vi "Text control 2 v3.1.vi"() -> ()   [LabVIEW 2016]
panel:
  out "I vs Vd":cluster{"Y data in":dbl[], "X data in":dbl[]}[](graph)
  in  "Auto Reset":bool
  in  "Reset":bool
  out "Id min vs time":cluster{"Y data in":dbl[], "X data in":dbl[]}[](graph)
  in  "Time Offset":dbl caption="Set Start Time (s)"
  out "Total lines":i32
  out "Line running":i32
  in  "byte count":u32=64
  in  "Serial Settings:Serial End Mode for Reads":u16(ring)=2 items=["None", "LastBit", "TermChar"]
  in  "Timeout (ms)":u32=10000
  in  "Enable Termination\nChar (T)":bool=TRUE
  in  "Termination char\n(0xA = '\\n' = LF)\n(0xD = '\\r' = CR)":u8=13 format="%.0x"
  in  "flow control":u16(ring) items=["None"=0, "XON/XOFF"=1, "RTS/CTS"=2, "DTR/DSR"=4]
  in  "stop bits":u16(ring)=10 items=["1.0"=10, "1.5"=15, "2.0"=20]
  in  "parity":u16(ring) items=["None", "Odd", "Even", "Mark", "Space"]
  in  "data bits":u16=8 min=5 max=8 step=1
  in  "VISA resource name":refnum<visa-resource-name>="COM6"
  in  "baud rate":u32=9600
  out "Serial port output":string
  out "error out":errorcluster
  in  "Units":u16(ring) items=["Seconds", "Minutes", "Hours"]
  out "Elapsed Time":dbl caption="Elapsed Time (s)"
  out "Id max vs time":cluster{"Y data in":dbl[], "X data in":dbl[]}[](graph)
  out "Ig":dbl format="%.2e"
  out "Id":dbl format="%.2e"
  out "Is":dbl format="%.2e"
  out "I vs Vg":cluster{"Y data in":dbl[], "X data in":dbl[]}[](graph)
  in  "Panel Controls 2":T1={"Emergency Stop"=refnum, "TransGraph Max"=1e-05, "Text/Graph (text=false)"=TRUE, "TransGraph Min"=1e-11} {"TransGraph Min" format="%.2e"; "TransGraph Max" format="%.2e"}
  out "Command running:":string="#output s 0 0 0 -0.008 0.008 0.002"
  in  "Standby":T2
  in  "Full Reset":bool
  in  "SMU4":cluster{"on/off":bool, "Voltage":dbl} {"Voltage" min=-100.0 max=100.0 format="%.2f"}
  in  "Source/Drain Range":u8(slide)=6 max=11 scale=0.0..11.0
  in  "Source/Drain\nRange mode":u16(ring) items=["Auto", "Limited", "Fixed"]
  in  "Gate Range":u8(slide)=6 max=11 scale=0.0..11.0
  in  "Gate Range\nmode":u16(ring) items=["Auto", "Limited", "Fixed"]
  in  "Gate":T3={"Gate Start"=0.0, "Gate Stop"=2.0, "Gate Step (linear only)"=1.0, "Gate Compliance"=0.0001, "Gate PComp"=0.0, "Range mode"=0, "Range"=6} {"Range" max=11 scale=0.0..11.0; "Range mode" items=["Auto", "Limited", "Fixed"]; "Gate PComp" format="%^.2e"; "Gate Compliance" format="%^.2e"; "Gate Step (linear only)" format="%^.4e"; "Gate Stop" format="%^.4e"; "Gate Start" format="%^.4e"}
  in  "Drain 2":T4={"Drain Start"=0.0, "Drain Stop"=2.0, "Drain Compliance"=0.0001, "Drain Step"=1.0, "Drain PComp"=0.0, "Range mode"=0, "Range"=6} {"Range" max=11 scale=0.0..11.0; "Range mode" items=["Auto", "Limited", "Fixed"]; "Drain PComp" format="%^.2e"; "Drain Step" format="%^.4e"; "Drain Compliance" format="%^.2e"; "Drain Stop" format="%^.4e"; "Drain Start" format="%^.4e"}
  in  "Timings 2":T5={"integration time"=0, "Short/Long integration time"=0.00064, "hold time (sec)"=0.0, "delay time (sec)"=0.0, "Step Time (0 disables)"=0.0, "sweep method"=0, "Pulse period"=0.005, "Base voltage"=0.0, "Pulse width"=0.0005} {"Pulse width" min=0.0005 max=0.1 step=0.0001 format="%.4f"; "Base voltage" format="%^.4e"; "Pulse period" min=0.005 max=1.0 step=0.0001 format="%.4f"; "sweep method" items=["Continuous", "Pulsed"]; "Step Time (0 disables)" format="%.2f"; "delay time (sec)" format="%.4f"; "hold time (sec)" format="%.4f"; "Short/Long integration time" format="%^.0e"; "integration time" scale=0.0..2.0}
  in  "Panel Controls":T6={"Emergency Stop"=refnum, "TransGraph Max"=1e-05, "Text/Graph (text=false)"=TRUE} {"TransGraph Max" format="%.2e"}
  in  "Interrupt run":bool
  in  "Drain: Compliance":dbl=0.001 format="%.8f"
  in  "Gate: Compliance":dbl=0.001 format="%.8f"
  out "Path":path=path "C:/users/rlp38/09Apr2009LTtesting/test2.txt"
  in  "hold time /s":dbl format="%.2f"
  in  "delay time /s":dbl format="%.2f"
  in  "integration time":u32(slide) max=2 step=1 scale=0.0..2.0
  in  "Integration time (short)":dbl=0.0019 min=8e-05 max=0.0019 step=8e-05 format="%^.0e"
  in  "Integration time (long)":dbl=0.32 min=0.04 max=2.0 step=0.02 format="%.2f"
  in  "Step delay /s":dbl format="%.2f"
  in  "Program":string="#pulsedstressV d 0.03 20 0 0.5 0.0827 5\n#\n#itime s\n#gaterangemode l\n#drainrangemode l\n#pulsed on 0.05 0 0.02\n#transfer d 1 -1 -0.1 -1 -1 0\n#wait-min 1\n#transfer d 1 -1 -0.1 -1 -1 0\n#output d 0 -1 -0.5 0 -1 -0.1\n#transfer d -10 40 1 5 40 35\n#transfer d -10 40 1 5 40 35\n#output d 0 40 20 0 40 1\n#\n#\n#sample 1 0.008 221 6 0.003\n#samplei 400e-6 200 6 0.002 0.1\n#vsu2pulse -10 4\n#\n#stressV 0.016 0.03 2e-4 0.1e-3 11\n#stressI 220e-7 0.08 15\n#transfer s -1 1 0.5 -0.005 0.005 0.005\n#output s 0 0 0 -0.008 0.008 0.002\n"
  # "Serial port settings"
  # "Time"
  # "100 samples is approx 13s with medium integration"
  # "Syntax:\nitime [s|m|l]\ngaterangemode [a|l|f]\ndrainrangemode [a|l|f]\npulsed [on|off] PulsePeriod(sec) PulseBaseVoltage PulseONWidth(sec)\nstandby [on l off]\nwait NumMilliseconds\nwait-min NumMinutes\n# texthere = comment\ntransfer [s|d] VgStart VgStop VgStep VdStart VdStop VdStep\noutput [s|d] VgStart VgStop VgStep VdStart VdStop VdStep\nsample Vg Vd NumSamples Time(s) SampleInterval(s)\nsamplei Idg NumSamples Time(s) SampleInterval(s) VDGcompliance\n# if in doubt use SampleInterval(s) = 0.004\nstressV VG VD IGcompliance IDcompliance Duration(sec)\nstressI IDG VDGcompliance Duration(sec)\nvsu2pulse Bias Duration(s)\npulsedstressV [s|d] VEstop VgON VgOFF Period(s) PulseONwidth(s) Vd\nsample-fpp Vg Vd NumSamples Time\nresample-fpp Vg Vd\ntransfer-fpp [s|d] VgStart VgStop VgStep VdStart VdStop VdStep\noutput-fpp [s|d] VgStart VgStop VgStep VdStart VdStop VdStep\nserial SerialPortCommand"
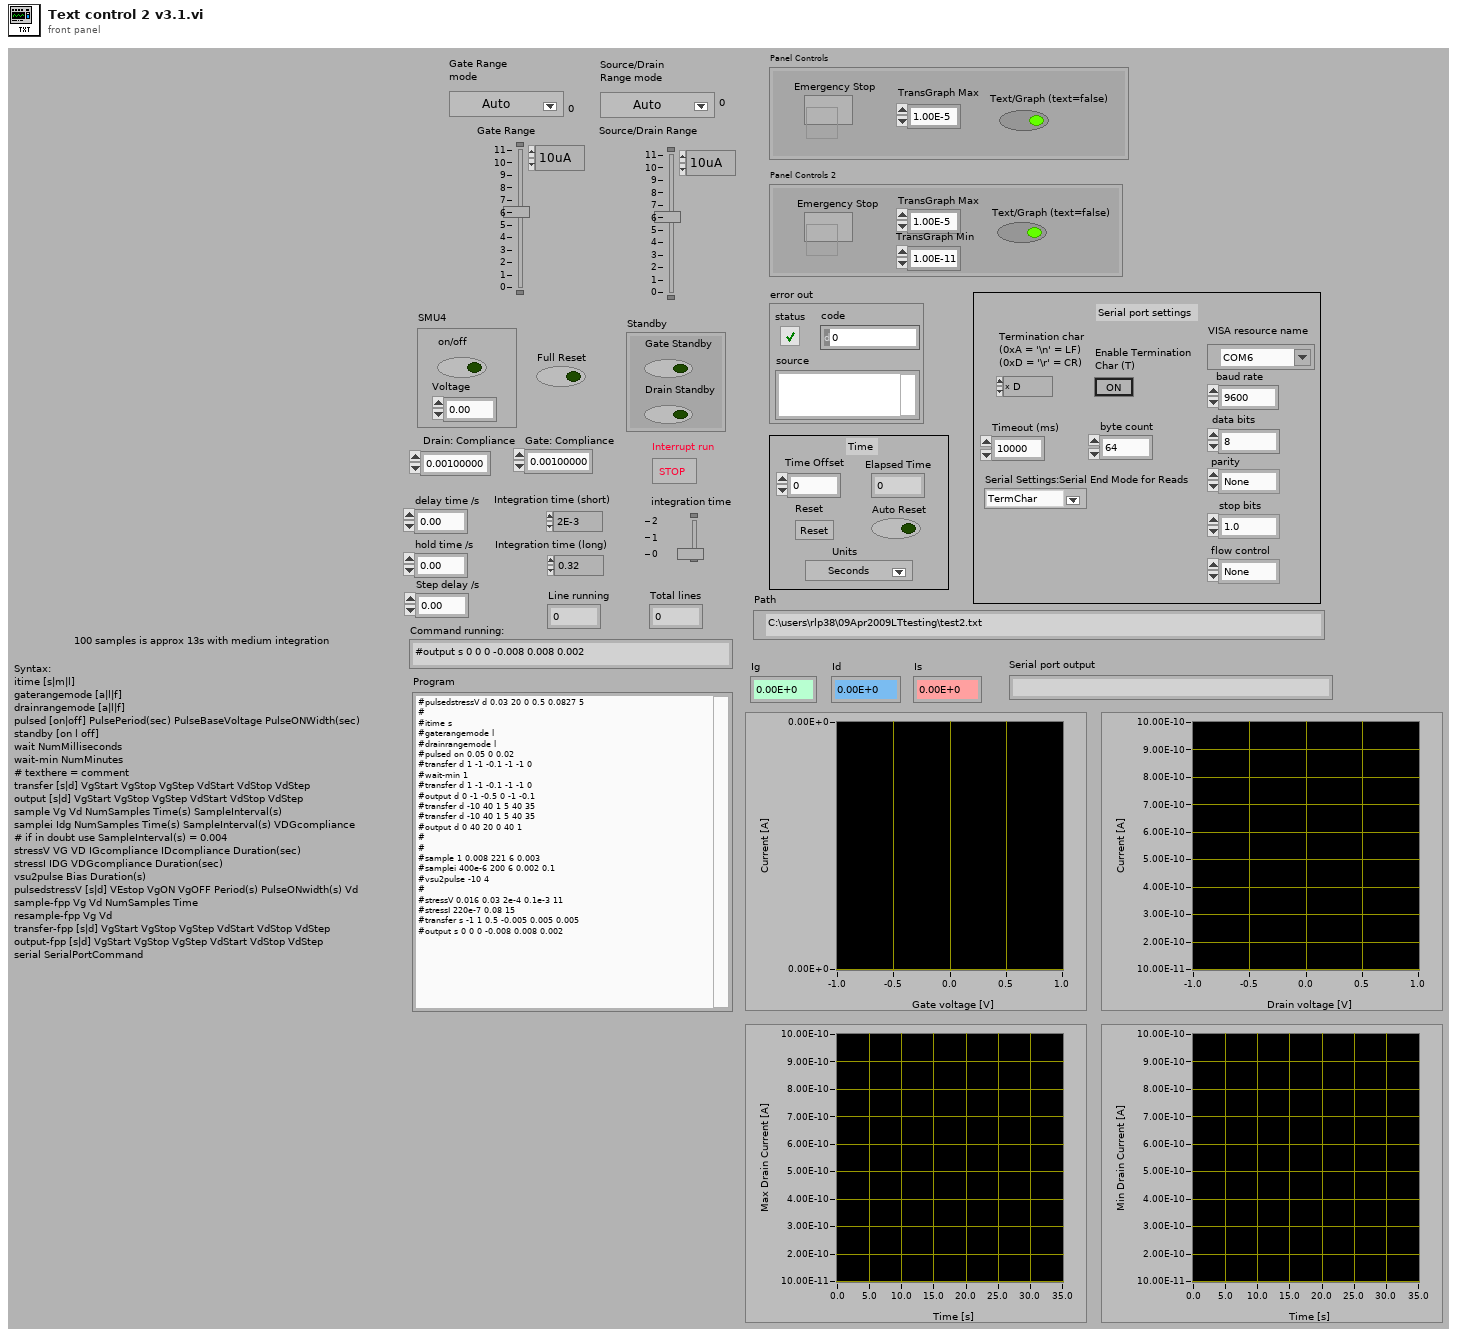
[diagram p1: front panel]
types:
  T1 = cluster{"Emergency Stop":refnum<vi>, "TransGraph Max":dbl, "Text/Graph (text=false)":bool, "TransGraph Min":dbl}
  T2 = cluster{"Gate Standby":bool, "Drain Standby":bool}
  T3 = cluster{"Gate Start":dbl, "Gate Stop":dbl, "Gate Step (linear only)":dbl, "Gate Compliance":dbl, "Gate PComp":dbl, "Range mode":u16, "Range":u8}
  T4 = cluster{"Drain Start":dbl, "Drain Stop":dbl, "Drain Compliance":dbl, "Drain Step":dbl, "Drain PComp":dbl, "Range mode":u16, "Range":u8}
  T5 = cluster{"integration time":u32, "Short/Long integration time":dbl, "hold time (sec)":dbl, "delay time (sec)":dbl, "Step Time (0 disables)":dbl, "sweep method":u16, "Pulse period":dbl, "Base voltage":dbl, "Pulse width":dbl}
  T6 = cluster{"Emergency Stop":refnum<vi>, "TransGraph Max":dbl, "Text/Graph (text=false)":bool}
  T7 = enum16{"open", "replace", "create", "open or create", "replace or create", "replace or create with confirmation"}
  T8 = cluster{"V2 Start":dbl, "V2 Step":dbl, "Number of points":i32}
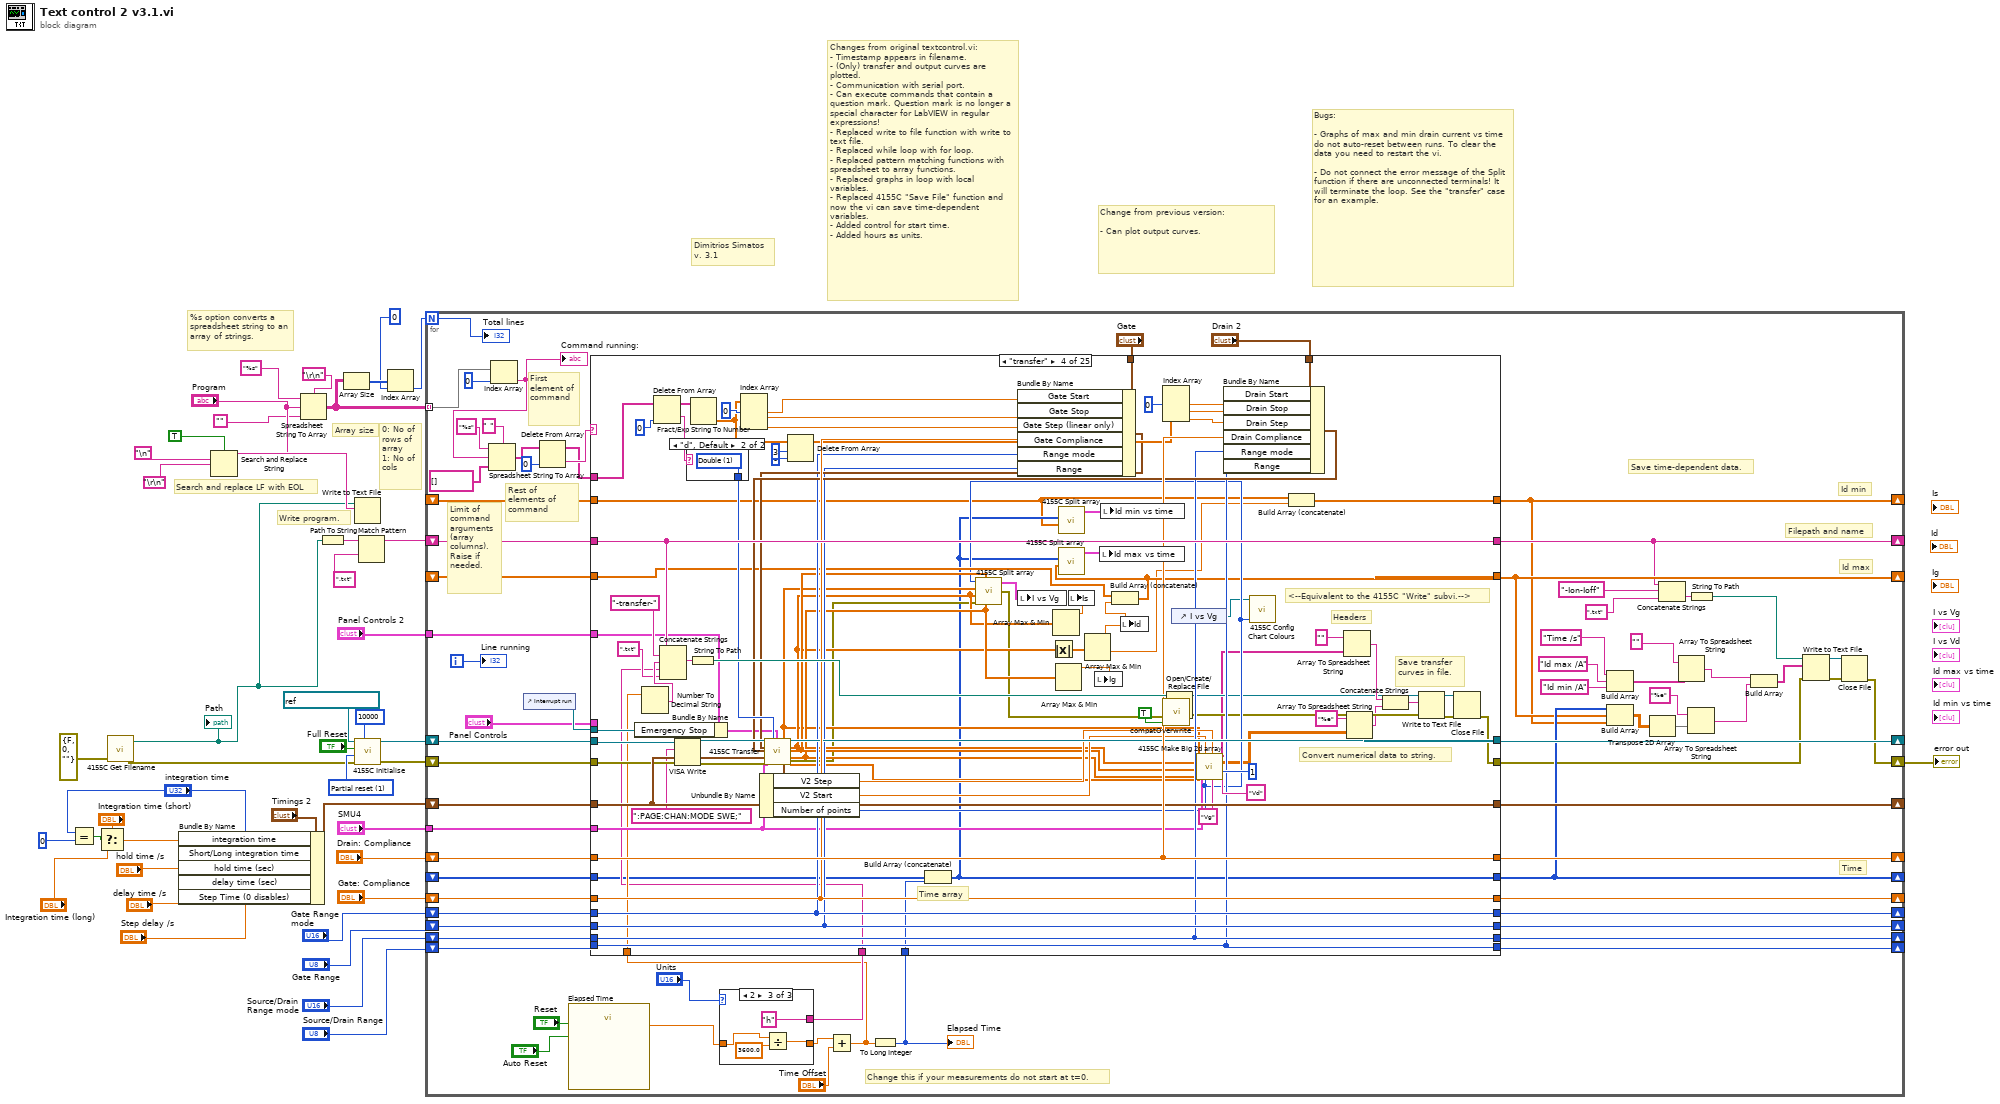
[diagram p0: block diagram]
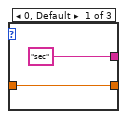
[diagram p2: hidden frame]
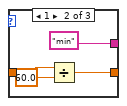
[diagram p3: hidden frame]
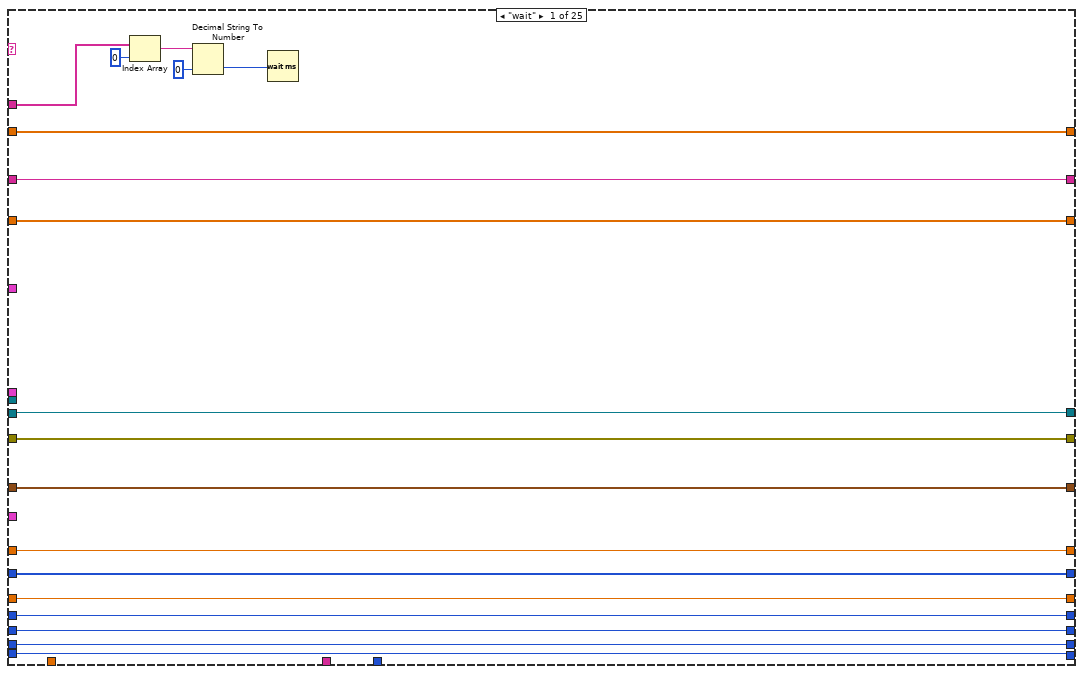
[diagram p4: hidden frame]
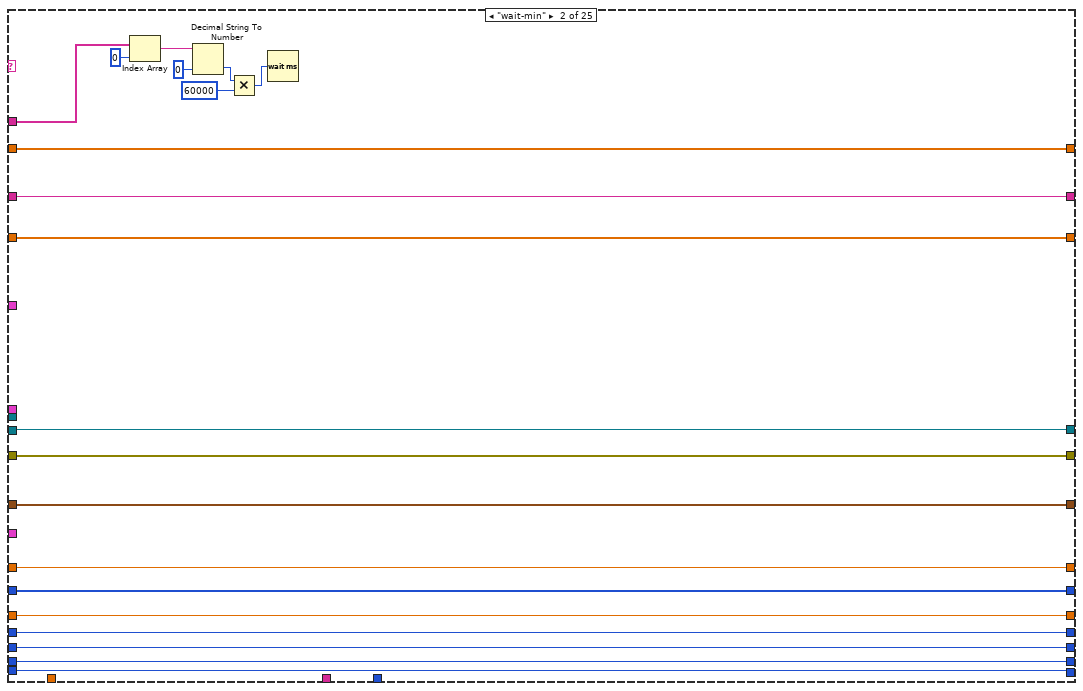
[diagram p5: hidden frame]
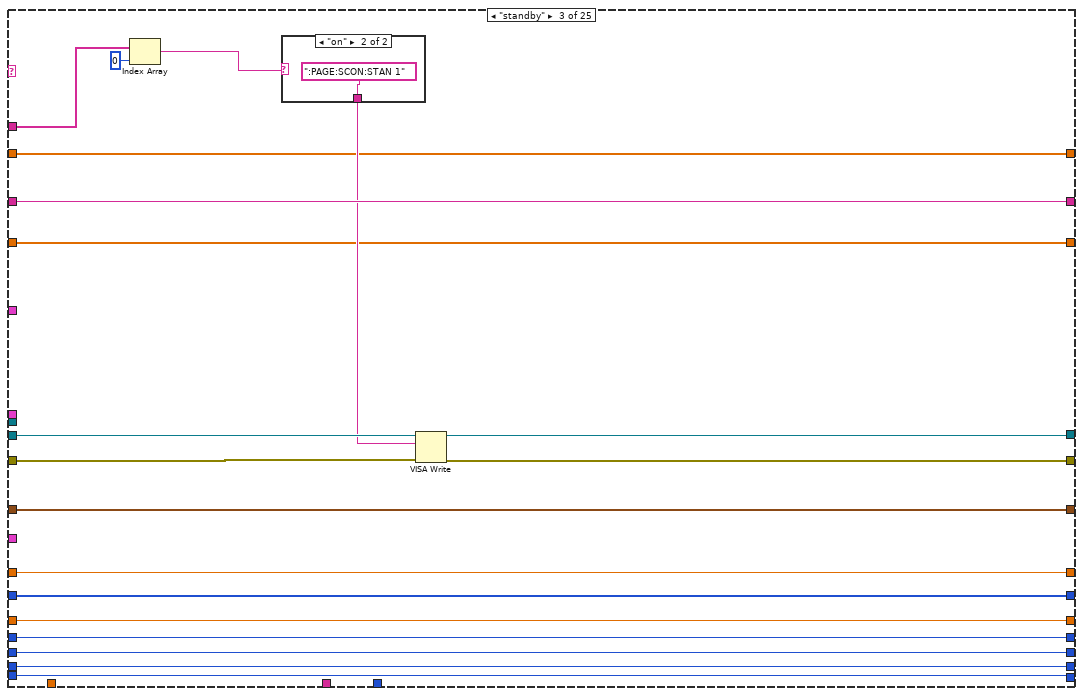
[diagram p6: hidden frame]
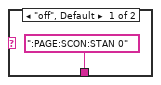
[diagram p7: hidden frame]
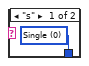
[diagram p8: hidden frame]
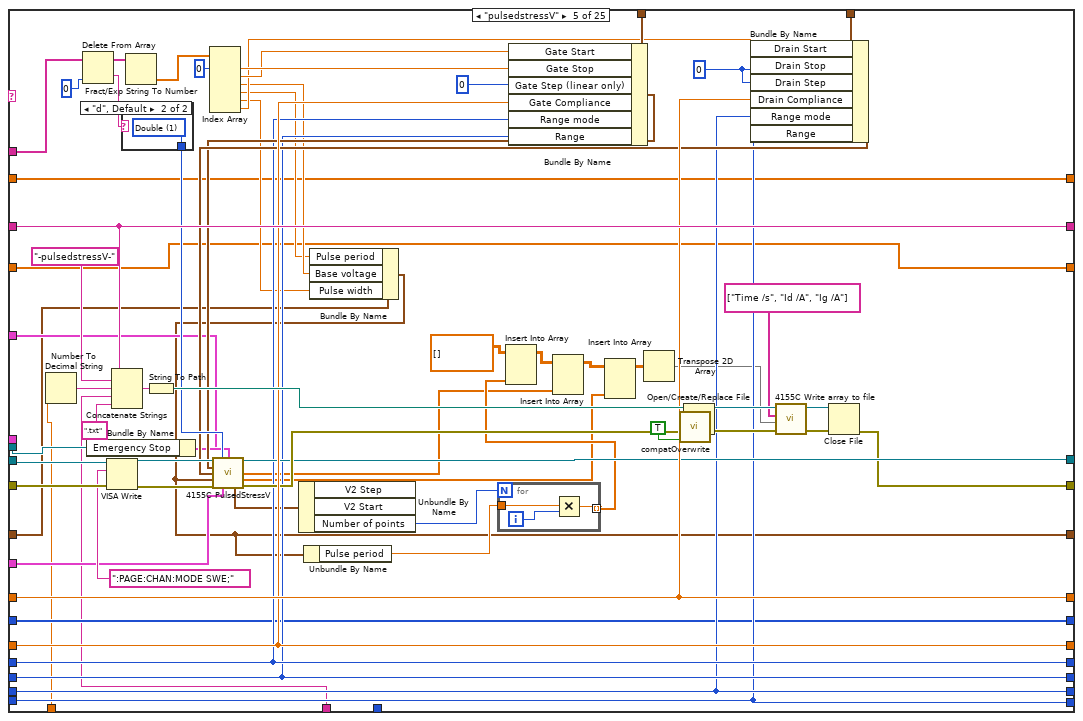
[diagram p9: hidden frame]
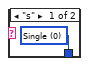
[diagram p10: hidden frame]
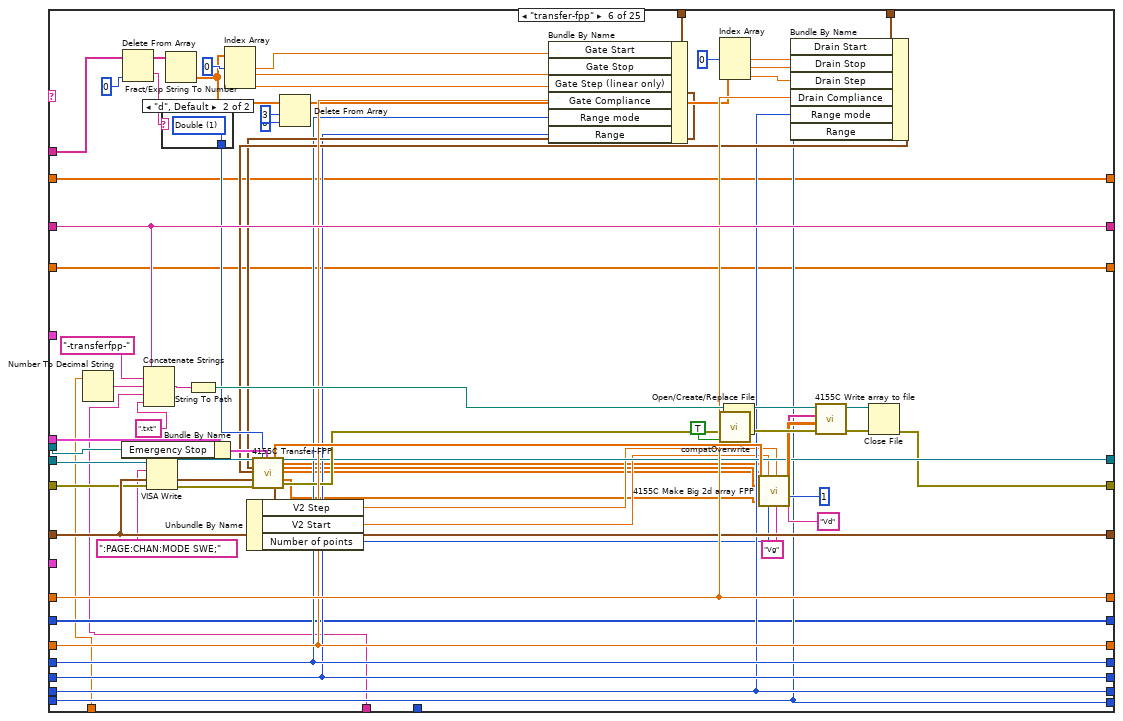
[diagram p11: hidden frame]
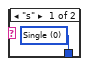
[diagram p12: hidden frame]
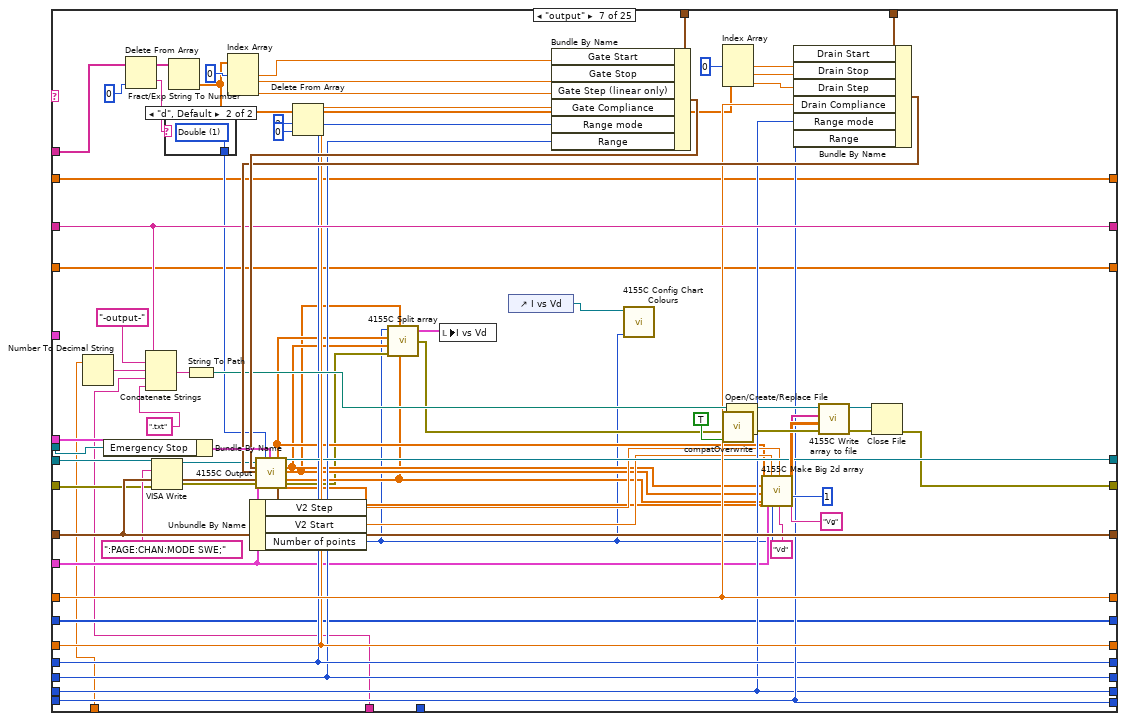
[diagram p13: hidden frame]
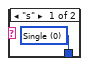
[diagram p14: hidden frame]
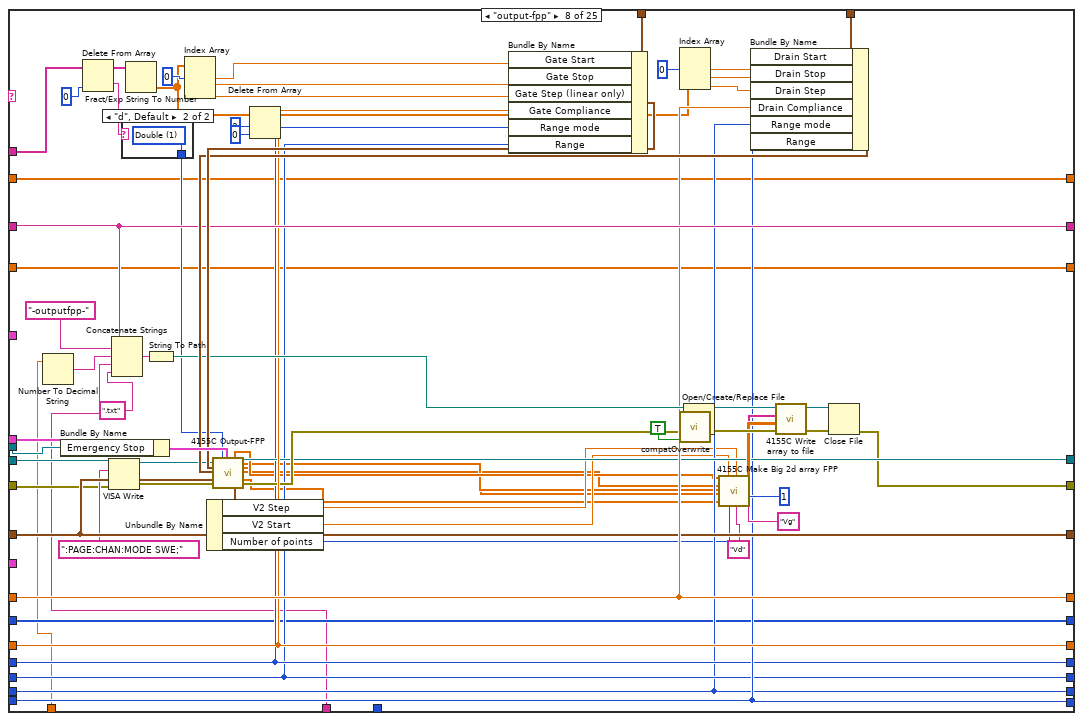
[diagram p15: hidden frame]
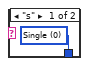
[diagram p16: hidden frame]
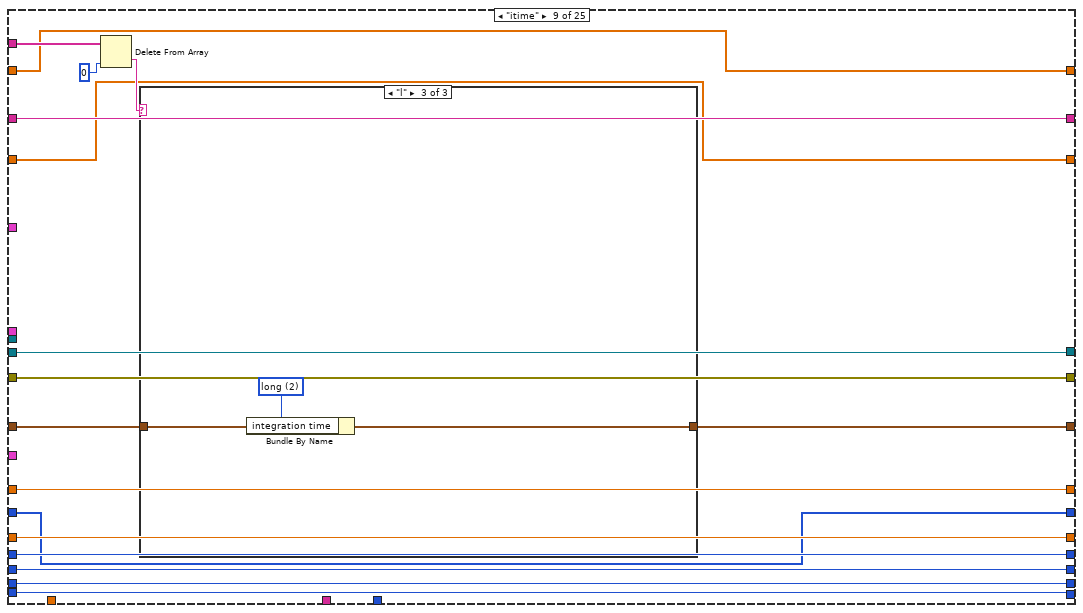
[diagram p17: hidden frame]
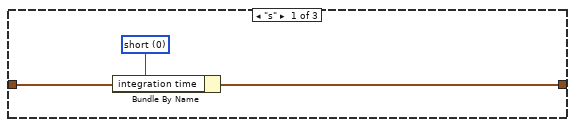
[diagram p18: hidden frame]
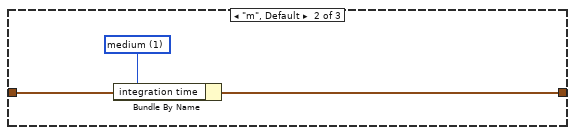
[diagram p19: hidden frame]
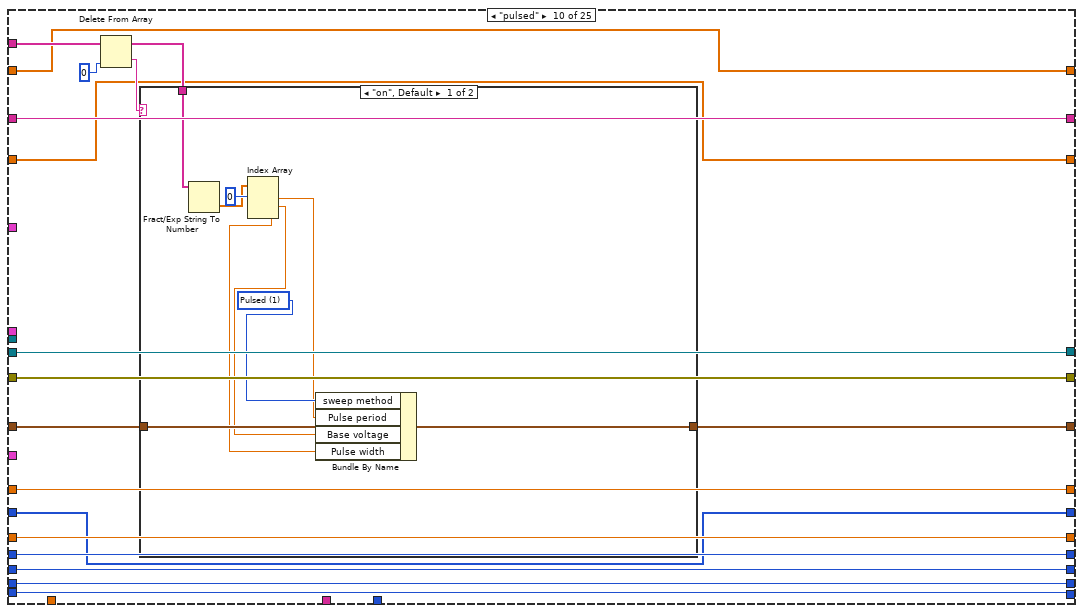
[diagram p20: hidden frame]
diagram:
  w35 = u16 1 items=["Reset All", "Partial reset"] ("Type of reset")
  # "Write program."
  # "Bugs:\n\n- Graphs of max and min drain current vs time do not auto-reset between runs. To clear the data you need to restart the vi.\n\n- Do not connect the error message of the Split function if there are unconnected terminals! It will terminate the loop. See the \"transfer\" case for an example."
  # "Array size"
  # "%s option converts a spreadsheet string to an array of strings."
  # "0: No of rows of array\n1: No of cols"
  # "Change from previous version:\n\n- Can plot output curves."
  # "Dimitrios Simatos\nv. 3.1"
  # "Changes from original textcontrol.vi:\n- Timestamp appears in filename.\n- (Only) transfer and output curves are plotted.\n- Communication with serial port.\n- Can execute commands that contain a question mark. Question mark is no longer a special character for LabVIEW in regular expressions!\n- Replaced write to file function with write to text file.\n- Replaced while loop with for loop.\n- Replaced pattern matching functions with spreadsheet to array functions.\n- Replaced graphs in loop with local variables.\n- Replaced 4155C \"Save File\" function and now the vi can save time-dependent variables.\n- Added control for start time.\n- Added hours as units."
  # "Search and replace LF with EOL"
  n1 = Equal?(x="integration time", y=u32 0) -> (x = y?=w39:bool)
  n2 = Select(t="Integration time (short)", s=w39, f="Integration time (long)") -> (s? t:f=w43:dbl)
  n3 = call "4155C Get Filename.vi"("error in (no error)"=errorcluster {"status"=FALSE, "code"=0, "source"=""}) -> ("error out"=w30:errorcluster, "path"=w2:path)  [unwired: 2 in, 1 out]
  "Path" <- w2
  n4 = Bundle By Name(cluster="Timings 2", "integration time"="integration time", "Short/Long integration time"=w43, "hold time (sec)"="hold time /s", "delay time (sec)"="delay time /s", "Step Time (0 disables)"="Step delay /s") -> (w27:T5)
  n5 = Search and Replace String(replace all?=TRUE ("replace all? (F)"), input string="Program", search string="\n", replace string="\r\n") -> (result string=w17:string)  [unwired: 4 in, 3 out]
  n6 = Spreadsheet String To Array(delimiter (Tab)="\r\n", format string="%s", spreadsheet string="Program", array type (2D Dbl)="") -> (array=w8:string[][])
  n7 = Path To String(path=w2) -> (string=w5:string)
  n8 = Array Size(array=w8) -> (size(s)=w12:i32[])
  n9 = Write to Text File(file (use dialog)=w2, text=w17) -> ()  [unwired: 2 in, 3 out]
  n10 = call "4155C Initialise.vi"("VISA resource name in"=refnum<visa-resource-name> "GPIB0::14::INSTR", "Reset"="Full Reset", "Type of reset"=w35, "error in (no error)"=w30, "VISA Timeout Value"=u32 10000) -> ("VISA Resource Name out"=w29:refnum<visa-resource-name>, "error out"=w28:errorcluster)
  n11 = Match Pattern(string=w5, regular expression=".txt") -> (before substring=w3:string)  [unwired: 1 in, 3 out]
  n12 = Index Array(array=w12, index=0) -> (element=w10:i32)
  n13 = for {
    N: w10 -> [w82]
    tunnel: "SMU4" -> [w93]
    shift-left: "Source/Drain Range" -> [w98]
    shift-right: [w94] -> _
    shift-left: "Source/Drain\nRange mode" -> [w99]
    shift-right: [w95] -> _
    shift-left: "Gate Range" -> [w100]
    shift-right: [w96] -> _
    shift-left: "Gate Range\nmode" -> [w101]
    shift-right: [w97] -> _
    shift-left: "Gate: Compliance" -> [w110]
    shift-right: [w106] -> _
    shift-left: "Drain: Compliance" -> [w111]
    shift-right: [w107] -> _
    shift-left: w27 -> [w112]
    shift-right: [w108] -> _
    shift-left: w28 -> [w113]
    shift-right: [w52] -> w1
    shift-left: w29 -> [w114]
    shift-right: [w109] -> _
    shift-left: w3 -> [w115]
    shift-right: [w55] -> _
    tunnel: "Panel Controls 2" -> [w92]
    shift-right: [w58] -> _
    shift-left: _ -> [w91]
    shift-right: [w59] -> _
    shift-left: _ -> [w87]
    tunnel: w8 -> [w85] mode=indexing
    shift-right: [w50] -> _
    shift-left: _ -> [w51]
    i -> [w83]
    # "Filepath and name"
    # "Save time-dependent data."
    # "Change this if your measurements do not start at t=0."
    # "Time"
    # "Rest of elements of command"
    # "Id min"
    # "Id max"
    # "Limit of command arguments (array columns). Raise if needed."
    # "First element of command"
    n14 = Index Array(array=w85, index=0 ("line index")) -> (element=w78:string)
    "Command running:" <- w78
    n15 = Spreadsheet String To Array(delimiter (Tab)=" ", format string="%s", spreadsheet string=w78, array type (2D Dbl)=string[] []) -> (array=w75:string[])
    n16 = control-ref of="Interrupt run"() -> (w105:refnum<vi>)
    n17 = Delete From Array(array=w75, index=0) -> (deleted portion=w76:string, array with subset deleted=w74:string[])  [unwired: 1 in]
    n18 = call "Elapsed Time"("Reset"="Reset", "Auto Reset"="Auto Reset") -> ("Elapsed Time (s)"=w88:dbl)  [unwired: 10 in, 7 out]
    n19 = case shown="2" "Units" {
      tunnel: ["sec" "min" "h"] -> w89
      tunnel: [w116 w120 w123] -> w46
      tunnel: w88 -> [w116 w119 w124]
      frame 0, Default {
      }
      frame 1 {
        n20 = Divide(x=w119, y=60.0) -> (x/y=w120:dbl)
      }
      frame 2 {
        n21 = Divide(x=w124, y=3600.0) -> (x/y=w123:dbl)
      }
    }
    n22 = Add(x=w46, y="Time Offset") -> (x+y=w45:dbl)
    n23 = To Long Integer(number=w45) -> (32bit integer=w86:i32)
    "Elapsed Time" <- w86
    n24 = case shown="\"transfer\"" w76 {
      tunnel: w74 -> [w143 w163 w182 w263 w328 w398 w474 w545 w584 w611 w639 w665 w687 w702 _ _ w809 w871 _ w938 w983 w1026 w1097 w1160 w1168]
      tunnel: w115 -> [w138 w159 w180 w270 w335 w406 w481 w553 w573 w600 w631 w658 w681 w695 w715 w758 w787 w853 w885 w925 w970 w1014 w1091 w1156 w1170]
      tunnel: w114 -> [w137 w158 w171 w241 w319 w375 w450 w521 w574 w601 w632 w659 w682 w696 w720 w760 w815 w877 w889 w944 w989 w1032 w1103 w1114 w1174]
      tunnel: w113 -> [w136 w157 w170 w240 w318 w374 w447 w518 w575 w602 w633 w660 w683 w697 w719 w731 w814 w876 w888 w943 w988 w1031 w1102 w1113 w1173]
      tunnel: w112 -> [w135 w156 w179 w266 w294 w402 w477 w549 w583 w610 w630 w657 w680 w694 w718 w755 w778 w845 w894 w918 w963 w1007 w1090 w1155 w1175]
      tunnel: w111 -> [w134 w155 w178 w268 w333 w404 w479 w551 w582 w609 w638 w664 w686 w701 w717 w740 w813 w875 w897 w942 w987 w1030 w1101 w1164 w1176]
      tunnel: w110 -> [w133 w154 w177 w267 w332 w403 w478 w550 w581 w608 w637 w663 w685 w700 w716 w741 w788 w854 w896 w926 w971 w1015 w1092 w1157 w1178]
      tunnel: [w137 w158 w169 w265 w330 w400 w476 w547 w574 w601 w632 w659 w682 w696 w720 w760 w779 w827 w887 w919 w964 w1008 w1043 w1116 w1174] -> w109
      tunnel: [w136 w157 w168 w264 w329 w399 w475 w546 w575 w602 w633 w660 w683 w697 w719 w730 w789 w828 w886 w927 w972 w1016 w1042 w1115 w1172] -> w53
      tunnel: [w135 w156 w179 w266 w290 w402 w477 w549 w576 w603 w630 w657 w680 w694 w718 w755 w778 w845 w894 w918 w963 w1007 w1090 w1155 w1175] -> w108
      tunnel: [w134 w155 w178 w268 w333 w404 w479 w551 w582 w609 w638 w664 w686 w701 w717 w740 w813 w875 w897 w942 w987 w1030 w1101 w1164 w1176] -> w107
      tunnel: [w133 w154 w177 w267 w332 w403 w478 w550 w581 w608 w637 w663 w685 w700 w716 w741 w788 w854 w896 w926 w971 w1015 w1092 w1157 w1178] -> w106
      tunnel: [w138 w159 w180 w270 w335 w406 w481 w553 w573 w600 w631 w658 w681 w695 w715 w758 w787 w853 w885 w925 w970 w1014 w1091 w1156 w1170] -> w55
      tunnel: w105 -> [_ _ _ w273 w339 w411 w485 w557 _ _ _ _ _ _ _ _ w784 w850 _ w924 w969 w1013 w1063 w1132 _]
      tunnel: "Gate" -> [_ _ _ w250 w322 w385 w461 w532 _ _ _ _ _ _ _ _ _ _ _ _ _ _ _ _ _]
      tunnel: "Drain 2" -> [_ _ _ w249 w321 w384 w460 w531 _ _ _ _ _ _ _ _ _ _ _ _ _ _ _ _ _]
      tunnel: "Panel Controls" -> [_ _ _ _ _ w383 w459 w530 _ _ _ _ _ _ _ _ _ _ _ _ _ _ _ _ _]
      tunnel: w101 -> [w132 w153 w176 w234 w312 w368 w445 w516 w580 w607 _ w656 w679 w693 w714 w742 w774 w841 w890 w914 w959 w1003 w1086 w1151 w1179]
      tunnel: w100 -> [w131 w152 w175 w233 w311 w367 w444 w515 w579 w606 w636 _ w670 w699 w713 w743 w775 w842 w891 w915 w960 w1004 w1087 w1152 w1180]
      tunnel: w99 -> [w130 w151 w174 w232 w310 w366 w443 w514 w578 w605 w635 w662 w684 _ w712 w744 w776 w843 w892 w916 w961 w1005 w1088 w1153 w1181]
      tunnel: w98 -> [w129 w150 w173 w231 w309 w365 w446 w517 w577 w604 w634 w661 _ w698 w711 w745 w777 w844 w893 w917 w962 w1006 w1089 w1154 w1182]
      tunnel: [w132 w153 w176 w234 w312 w368 w445 w516 w580 w607 w629 w656 w679 w693 w714 w742 w774 w841 w890 w914 w959 w1003 w1086 w1151 w1179] -> w97
      tunnel: [w131 w152 w175 w233 w311 w367 w444 w515 w579 w606 w636 w648 w670 w699 w713 w743 w775 w842 w891 w915 w960 w1004 w1087 w1152 w1180] -> w96
      tunnel: [w130 w151 w174 w232 w310 w366 w443 w514 w578 w605 w635 w662 w684 w692 w712 w744 w776 w843 w892 w916 w961 w1005 w1088 w1153 w1181] -> w95
      tunnel: [w129 w150 w173 w231 w309 w365 w446 w517 w577 w604 w634 w661 w671 w698 w711 w745 w777 w844 w893 w917 w962 w1006 w1089 w1154 w1182] -> w94
      tunnel: w93 -> [_ _ _ w226 w306 _ w439 _ _ _ _ _ _ _ _ _ _ _ _ _ _ _ _ _ _]
      tunnel: w92 -> [_ _ _ w224 w305 _ _ _ _ _ _ _ _ _ _ _ _ _ _ _ _ _ _ _ _]
      tunnel: [w128 w146 w166 w192 w282 w355 w436 w503 w572 w598 w628 w647 w669 w691 w710 w726 w766 w825 w884 w903 w952 w997 w1040 w1109 w1171] -> w58
      tunnel: w91 -> [w128 w146 w166 w215 w282 w355 w436 w503 w572 w598 w628 w647 w669 w691 w710 w726 w766 w825 w884 w903 w952 w997 w1040 w1109 w1171]
      tunnel: w45 -> [_ _ _ w211 w279 w353 w433 w500 _ _ _ _ _ _ _ w724 w764 w822 _ w900 w949 w994 w1037 w1105 _]
      tunnel: w89 -> [_ _ _ w208 w278 w351 w432 w499 _ _ _ _ _ _ _ w722 w762 w821 _ w899 w948 w993 w1036 w1106 _]
      tunnel: w86 -> [_ _ _ w193 _ _ _ _ _ _ _ _ _ _ _ _ _ _ _ _ _ _ _ _ _]
      tunnel: [w127 w145 w165 w188 w281 w354 w435 w502 w571 w597 w627 w646 w668 w690 w709 w725 w765 w824 w883 w902 w951 w996 w1039 w1108 w1177] -> w59
      tunnel: w87 -> [w127 w145 w165 w207 w281 w354 w435 w502 w571 w597 w627 w646 w668 w690 w709 w725 w765 w824 w883 w902 w951 w996 w1039 w1108 w1177]
      tunnel: [w126 w144 w164 w186 w277 w350 w431 w498 w570 w596 w626 w645 w667 w689 w708 w721 w761 w820 w882 w898 w947 w992 w1035 w1104 w1165] -> w50
      tunnel: w51 -> [w126 w144 w164 w185 w277 w350 w431 w498 w570 w596 w626 w645 w667 w689 w708 w721 w761 w820 w882 w898 w947 w992 w1035 w1104 w1165]
      frame "wait" {
        n25 = Index Array(array=w143, index=0 ("Index")) -> (element=w141:string)
        n26 = Decimal String To Number(string=w141, default (0L)=u32 0) -> (number=w140:u32)  [unwired: 1 in, 1 out]
        n27 = Wait (ms)(milliseconds to wait=w140) -> ()  [unwired: 1 out]
      }
      frame "wait-min" {
        n28 = Index Array(array=w163, index=0 ("Index")) -> (element=w161:string)
        n29 = Decimal String To Number(string=w161, default (0L)=u32 0) -> (number=w149:u32)  [unwired: 1 in, 1 out]
        n30 = Multiply(x=w149, y=u32 60000) -> (x*y=w148:u32)
        n31 = Wait (ms)(milliseconds to wait=w148) -> ()  [unwired: 1 out]
      }
      frame "standby" {
        n32 = Index Array(array=w182, index=0 ("Index")) -> (element=w172:string)
        n33 = case shown="\"on\"" w172 {
          tunnel: [":PAGE:SCON:STAN 0" ":PAGE:SCON:STAN 1"] -> w167
          frame "off", Default {
          }
          frame "on" {
          }
        }
        n34 = VISA Write(VISA resource name=w171, write buffer=w167, error in (no error)=w170) -> (VISA resource name out=w169:refnum<visa-resource-name>, error out=w168:errorcluster)  [unwired: 1 out]
      }
      frame "transfer" {
        # "<--Equivalent to the 4155C \"Write\" subvi.-->"
        # "Headers"
        # "Convert numerical data to string."
        # "Save transfer curves in file."
        # "Time array"
        n35 = Bundle By Name(cluster=w224, "Emergency Stop"=w273) -> (w225:T1)
        n36 = Number To Decimal String(number=w211) -> (decimal integer string=w210:string)  [unwired: 1 in]
        n37 = Delete From Array(array=w263, index=0 ("Index")) -> (deleted portion=w261:string, array with subset deleted=w260:string[])  [unwired: 1 in]
        n38 = Concatenate Strings(w270, "-transfer-" ("Prefix"), w210, w208, ".txt" ("Suffix")) -> (w272:string)
        n39 = VISA Write(VISA resource name=w241, write buffer=":PAGE:CHAN:MODE SWE;" ("write buffer (\"\")"), error in (no error)=w240) -> (VISA resource name out=w238:refnum<visa-resource-name>, error out=w239:errorcluster)  [unwired: 1 out]
        n40 = case shown="\"d\", Default" w261 {
          tunnel: [w275 w276] -> w259
          frame "s" {
            w275 = u16 0 items=["Single", "Double"] ("sweep mode")
          }
          frame "d", Default {
            w276 = u16 1 items=["Single", "Double"] ("sweep mode")
          }
        }
        n41 = String To Path(string=w272) -> (path=w269:path)
        n42 = Fract/Exp String To Number(string=w260) -> (number=w245:dbl[])  [unwired: 3 in, 1 out]
        n43 = Index Array(array=w245, index #1=0 ("Index")) -> (element #1=w258:dbl, element #2=w257:dbl, element #3=w256:dbl)  [unwired: 2 in]
        n44 = Delete From Array(array=w245, length=3 ("Length"), index=0 ("Index")) -> (array with subset deleted=w243:dbl[])  [unwired: 1 out]
        n45 = Build Array (concatenate)(w207, w193) -> (w188:i32[])
        n46 = Bundle By Name(cluster=w250, "Gate Start"=w258, "Gate Stop"=w257, "Gate Step (linear only)"=w256, "Gate Compliance"=w267, "Range mode"=w234, "Range"=w233) -> (w235:T3)
        n47 = call "4155C Split array.vi"("X data in"=w188, "Y1 data in"=w185) -> ("Array of clusters"=w189:cluster{"Y data in":dbl[], "X data in":dbl[]}[])  [unwired: 5 in, 1 out]
        n48 = local write "Id min vs time"(w189) -> ()
        n49 = Index Array(array=w243, index #1=0 ("Index")) -> (element #1=w253:dbl, element #2=w252:dbl, element #3=w251:dbl)  [unwired: 2 in]
        n50 = call <vilib>:"compatOverwrite.vi"("overwrite (F)"=TRUE) -> ("overwrite?"=w223:T7)
        n51 = control-ref of="I vs Vg"() -> (w212:refnum<vi>)
        n52 = Bundle By Name(cluster=w249, "Drain Start"=w253, "Drain Stop"=w252, "Drain Step"=w251, "Drain Compliance"=w268, "Range mode"=w232, "Range"=w231) -> (w236:T4)
        n53 = call "4155C Transfer.vi"("VISA resource name in"=w238, "Gate"=w235, "Drain"=w236, "Timings"=w266, "error in (no error)"=w239, "SMU4"=w226, "sweep mode"=w259, "Panel Controls"=w225) -> ("VG"=w216:dbl[], "Outparams"=w230:T8, "VISA Resource Name out"=w265:refnum<visa-resource-name>, "IS"=w217:dbl[], "ID"=w222:dbl[], "IG"=w218:dbl[], "error out"=w203:errorcluster, "SMU4"=w227:dbl[])  [unwired: 12 in]
        n54 = Unbundle By Name(w230) -> ("V2 Step"=w229:dbl, "V2 Start"=w228:dbl, "Number of points"=w213:i32)
        n55 = call "4155C Split array.vi"("Number of VAR2 steps"=w213, "Y2 data in"=w222, "X data in"=w216, "Y1 data in"=w217, "Y3 data in"=w218, "error in (no error)"=w203) -> ("Array of clusters"=w206:cluster{"Y data in":dbl[], "X data in":dbl[]}[], "error out"=w204:errorcluster)  [unwired: 1 in]
        n56 = local write "I vs Vg"(w206) -> ()
        n57 = Absolute Value(x=w217) -> (abs(x)=w221:dbl[])
        n58 = Array Max & Min(array=w217) -> (max value=w219:dbl)  [unwired: 3 out]
        n59 = Array Max & Min(array=w218) -> (max value=w220:dbl)  [unwired: 3 out]
        n60 = local write "Is"(w219) -> ()
        n61 = Array Max & Min(array=w221) -> (max value=w214:dbl, min value=w187:dbl)  [unwired: 2 out]
        n62 = local write "Ig"(w220) -> ()
        n63 = Build Array (concatenate)(w215, w214) -> (w192:dbl[])
        n64 = call "4155C Split array.vi"("X data in"=w188, "Y1 data in"=w192) -> ("Array of clusters"=w205:cluster{"Y data in":dbl[], "X data in":dbl[]}[])  [unwired: 5 in, 1 out]
        n65 = local write "Id max vs time"(w205) -> ()
        n66 = local write "Id"(w214) -> ()
        n67 = Open/Create/Replace File(file path (use dialog)=w269, error in=w204, operation (0:open)=w223) -> (refnum out=w191:refnum<file>, error out=w200:errorcluster)  [unwired: 3 in, 1 out]
        n68 = call "4155C Make Big 2d array.vi"("1D Var1"=w216, "1d IS"=w217, "1d ID"=w222, "1d IG"=w218, "1d SMU4"=w227, "SMU4"=w226, "VAR2 START"=w228, "Number of VAR2 steps"=w213, "VAR2 STEP"=w229, "VAR1 Name"="Vg", "Decimal places in header"=i8 1, "VAR2 Name"="Vd") -> ("Header array"=w190:string[], "Data array"=w197:dbl[][])  [unwired: 14 in]
        n69 = call "4155C Config Chart Colours.vi"("Numeric"=w213, "XY Graph 2"=w212) -> ()  [unwired: 6 in]
        n70 = Build Array (concatenate)(w185, w187) -> (w186:dbl[])
        n71 = Array To Spreadsheet String(array=w190, 3:"" ("format string")) -> (spreadsheet string=w196:string)  [unwired: 1 in]
        n72 = Array To Spreadsheet String(array=w197, 3:"%e" ("format string")) -> (spreadsheet string=w199:string)  [unwired: 1 in]
        n73 = Concatenate Strings(w196, w199) -> (w198:string)
        n74 = Write to Text File(file (use dialog)=w191, text=w198, error in=w200) -> (refnum out=w202:refnum<file>, error out=w201:errorcluster)  [unwired: 1 in, 1 out]
        n75 = Close File(refnum=w202, error in=w201) -> (error out=w264:errorcluster)  [unwired: 1 out]
      }
      frame "pulsedstressV" {
        w288 = 0
        n76 = Number To Decimal String(number=w279) -> (decimal integer string=w336:string)  [unwired: 1 in]
        n77 = Delete From Array(array=w328, index=0 ("Index")) -> (deleted portion=w326:string, array with subset deleted=w325:string[])  [unwired: 1 in]
        n78 = Bundle By Name(cluster=w305, "Emergency Stop"=w339) -> (w307:T1)
        n79 = VISA Write(VISA resource name=w319, write buffer=":PAGE:CHAN:MODE SWE;" ("write buffer (\"\")"), error in (no error)=w318) -> (VISA resource name out=w316:refnum<visa-resource-name>, error out=w317:errorcluster)  [unwired: 1 out]
        n80 = Concatenate Strings(w335, "-pulsedstressV-" ("Substring"), w336, w278, ".txt" ("Substring")) -> (w338:string)
        n81 = case shown="\"d\", Default" w326 {
          tunnel: [w348 w349] -> w324
          frame "s" {
            w348 = u16 0 items=["Single", "Double"] ("sweep mode")
          }
          frame "d", Default {
            w349 = u16 1 items=["Single", "Double"] ("sweep mode")
          }
        }
        n82 = Fract/Exp String To Number(string=w325) -> (number=w320:dbl[])  [unwired: 3 in, 1 out]
        n83 = String To Path(string=w338) -> (path=w334:path)
        n84 = Index Array(array=w320, index #1=0 ("Index")) -> (element #1=w297:dbl, element #2=w296:dbl, element #3=w293:dbl, element #4=w292:dbl, element #5=w291:dbl, element #6=w295:dbl)  [unwired: 5 in]
        n85 = Bundle By Name(cluster=w294, "Pulse period"=w292, "Base voltage"=w293, "Pulse width"=w291) -> (w290:T5)
        n86 = Unbundle By Name(w290) -> ("Pulse period"=w298:dbl)
        n87 = Bundle By Name(cluster=w322, "Gate Start"=w296, "Gate Stop"=w297, "Gate Step (linear only)"=0, "Gate Compliance"=w332, "Range mode"=w312, "Range"=w311) -> (w313:T3)
        n88 = call <vilib>:"compatOverwrite.vi"("overwrite (F)"=TRUE) -> ("overwrite?"=w283:T7)
        n89 = Bundle By Name(cluster=w321, "Drain Start"=w295, "Drain Stop"=w288, "Drain Step"=w288, "Drain Compliance"=w333, "Range mode"=w310, "Range"=w309) -> (w314:T4)
        n90 = call "4155C PulsedStressV.vi"("VISA resource name in"=w316, "sweep mode"=w324, "Panel Controls"=w307, "Gate"=w313, "Drain"=w314, "Timings"=w290, "error in (no error)"=w317, "SMU4"=w306) -> ("VISA Resource Name out"=w330:refnum<visa-resource-name>, "ID"=w286:dbl[], "IG"=w284:dbl[], "Outparams"=w308:T8, "error out"=w331:errorcluster)  [unwired: 3 in]
        n91 = Unbundle By Name(w308) -> ("Number of points"=w285:i32)  [unwired: 2 out]
        n92 = for {
          N: w285 -> [_]
          tunnel: [w345] -> w287 mode=indexing
          tunnel: w298 -> [w347]
          i -> [w346]
          n93 = Multiply(x=w347, y=w346) -> (x*y=w345:dbl)
        }
        n94 = Insert Into Array(array=dbl[][] [] ("Input Array"), new element=w287) -> (w299:dbl[][])  [unwired: 2 in]
        n95 = Insert Into Array(array=w299, new element=w286) -> (w304:dbl[][])  [unwired: 2 in]
        n96 = Insert Into Array(array=w304, new element=w284) -> (w303:dbl[][])  [unwired: 2 in]
        n97 = Transpose 2D Array(2D array=w303) -> (transposed array=w302:dbl[][])
        n98 = Open/Create/Replace File(file path (use dialog)=w334, error in=w331, operation (0:open)=w283) -> (refnum out=w342:refnum<file>, error out=w343:errorcluster)  [unwired: 3 in, 1 out]
        n99 = call "4155C Write array to file.vi"("Byte Stream File Refnum"=w342, "Header"=string[] ["Time /s", "Id /A", "Ig /A"], "Data Array"=w302, "error in (no error)"=w343) -> ("dup refnum"=w340:refnum<file>, "error out"=w341:errorcluster)  [unwired: 1 in]
        n100 = Close File(refnum=w340, error in=w341) -> (error out=w329:errorcluster)  [unwired: 1 out]
      }
      frame "transfer-fpp" {
        n101 = Number To Decimal String(number=w353) -> (decimal integer string=w407:string)  [unwired: 1 in]
        n102 = Bundle By Name(cluster=w383, "Emergency Stop"=w411) -> (w419:T6)
        n103 = Delete From Array(array=w398, index=0 ("Index")) -> (deleted portion=w396:string, array with subset deleted=w395:string[])  [unwired: 1 in]
        n104 = Concatenate Strings(w406, "-transferfpp-" ("Substring"), w407, w351, ".txt" ("Substring")) -> (w409:string)
        n105 = VISA Write(VISA resource name=w375, write buffer=":PAGE:CHAN:MODE SWE;" ("write buffer (\"\")"), error in (no error)=w374) -> (VISA resource name out=w372:refnum<visa-resource-name>, error out=w373:errorcluster)  [unwired: 1 out]
        n106 = case shown="\"d\", Default" w396 {
          tunnel: [w420 w421] -> w394
          frame "s" {
            w420 = u16 0 items=["Single", "Double"] ("sweep mode")
          }
          frame "d", Default {
            w421 = u16 1 items=["Single", "Double"] ("sweep mode")
          }
        }
        n107 = Fract/Exp String To Number(string=w395) -> (number=w379:dbl[])  [unwired: 3 in, 1 out]
        n108 = String To Path(string=w409) -> (path=w405:path)
        n109 = Index Array(array=w379, index #1=0 ("Index")) -> (element #1=w393:dbl, element #2=w392:dbl, element #3=w391:dbl)  [unwired: 2 in]
        n110 = Delete From Array(array=w379, length=3 ("Length"), index=0 ("Index")) -> (array with subset deleted=w377:dbl[])  [unwired: 1 out]
        n111 = Bundle By Name(cluster=w385, "Gate Start"=w393, "Gate Stop"=w392, "Gate Step (linear only)"=w391, "Gate Compliance"=w403, "Range mode"=w368, "Range"=w367) -> (w369:T3)
        n112 = Index Array(array=w377, index #1=0 ("Index")) -> (element #1=w388:dbl, element #2=w387:dbl, element #3=w386:dbl)  [unwired: 2 in]
        n113 = call <vilib>:"compatOverwrite.vi"("overwrite (F)"=TRUE) -> ("overwrite?"=w356:T7)
        n114 = Bundle By Name(cluster=w384, "Drain Start"=w388, "Drain Stop"=w387, "Drain Step"=w386, "Drain Compliance"=w404, "Range mode"=w366, "Range"=w365) -> (w370:T4)
        n115 = call "4155C Transfer-FPP.vi"("VISA resource name in"=w372, "Gate"=w369, "Drain"=w370, "Timings"=w402, "error in (no error)"=w373, "sweep mode"=w394, "Panel Controls"=w419) -> ("VG"=w410:dbl[], "Outparams"=w364:T8, "VISA Resource Name out"=w400:refnum<visa-resource-name>, "Vprobe2"=w360:dbl[], "ID"=w359:dbl[], "IG"=w358:dbl[], "Vprobe1"=w357:dbl[], "error out"=w401:errorcluster)  [unwired: 13 in]
        n116 = Unbundle By Name(w364) -> ("V2 Step"=w363:dbl, "V2 Start"=w362:dbl, "Number of points"=w361:i32)
        n117 = Open/Create/Replace File(file path (use dialog)=w405, error in=w401, operation (0:open)=w356) -> (refnum out=w416:refnum<file>, error out=w417:errorcluster)  [unwired: 3 in, 1 out]
        n118 = call "4155C Make Big 2d array FPP.vi"("1D Var1"=w410, "1d ID"=w359, "1d Vp2"=w360, "1d IG"=w358, "1d Vp1"=w357, "VAR2 START"=w362, "Number of VAR2 steps"=w361, "VAR2 STEP"=w363, "VAR1 Name"="Vg", "Decimal places in header"=i8 1, "VAR2 Name"="Vd") -> ("Header array"=w412:string[], "Data array"=w413:dbl[][])  [unwired: 15 in]
        n119 = call "4155C Write array to file.vi"("Byte Stream File Refnum"=w416, "Header"=w412, "Data Array"=w413, "error in (no error)"=w417) -> ("dup refnum"=w414:refnum<file>, "error out"=w415:errorcluster)  [unwired: 1 in]
        n120 = Close File(refnum=w414, error in=w415) -> (error out=w399:errorcluster)  [unwired: 1 out]
      }
      frame "output" {
        n121 = Number To Decimal String(number=w433) -> (decimal integer string=w482:string)  [unwired: 1 in]
        n122 = Bundle By Name(cluster=w459, "Emergency Stop"=w485) -> (w495:T6)
        n123 = Delete From Array(array=w474, index=0 ("Index")) -> (deleted portion=w472:string, array with subset deleted=w471:string[])  [unwired: 1 in]
        n124 = Concatenate Strings(w481, "-output-" ("Substring"), w482, w432, ".txt" ("Substring")) -> (w484:string)
        n125 = VISA Write(VISA resource name=w450, write buffer=":PAGE:CHAN:MODE SWE;" ("write buffer (\"\")"), error in (no error)=w447) -> (VISA resource name out=w449:refnum<visa-resource-name>, error out=w448:errorcluster)  [unwired: 1 out]
        n126 = case shown="\"d\", Default" w472 {
          tunnel: [w496 w497] -> w470
          frame "s" {
            w496 = u16 0 items=["Single", "Double"] ("sweep mode")
          }
          frame "d", Default {
            w497 = u16 1 items=["Single", "Double"] ("sweep mode")
          }
        }
        n127 = Fract/Exp String To Number(string=w471) -> (number=w453:dbl[])  [unwired: 3 in, 1 out]
        n128 = String To Path(string=w484) -> (path=w480:path)
        n129 = Index Array(array=w453, index #1=0 ("Index")) -> (element #1=w469:dbl, element #2=w468:dbl, element #3=w467:dbl)  [unwired: 2 in]
        n130 = Delete From Array(array=w453, length=3 ("Length"), index=0 ("Index")) -> (array with subset deleted=w452:dbl[])  [unwired: 1 out]
        n131 = control-ref of="I vs Vd"() -> (w423:refnum<vi>)
        n132 = Bundle By Name(cluster=w461, "Gate Start"=w469, "Gate Stop"=w468, "Gate Step (linear only)"=w467, "Gate Compliance"=w478, "Range mode"=w445, "Range"=w444) -> (w494:T3)
        n133 = Index Array(array=w452, index #1=0 ("Index")) -> (element #1=w464:dbl, element #2=w463:dbl, element #3=w462:dbl)  [unwired: 2 in]
        n134 = call <vilib>:"compatOverwrite.vi"("overwrite (F)"=TRUE) -> ("overwrite?"=w437:T7)
        n135 = Bundle By Name(cluster=w460, "Drain Start"=w464, "Drain Stop"=w463, "Drain Step"=w462, "Drain Compliance"=w479, "Range mode"=w443, "Range"=w446) -> (w493:T4)
        n136 = call "4155C Output.vi"("VISA resource name in"=w449, "Gate"=w494, "Drain"=w493, "Timings"=w477, "error in (no error)"=w448, "SMU4"=w439, "sweep mode"=w470, "Panel controls"=w495) -> ("VD"=w430:dbl[], "Outparams"=w441:T8, "VISA Resource Name out"=w476:refnum<visa-resource-name>, "IS"=w429:dbl[], "ID"=w428:dbl[], "IG"=w427:dbl[], "error out"=w425:errorcluster, "SMU4"=w438:dbl[])  [unwired: 12 in]
        n137 = Unbundle By Name(w441) -> ("V2 Step"=w442:dbl, "V2 Start"=w440:dbl, "Number of points"=w422:i32)
        n138 = call "4155C Split array.vi"("Number of VAR2 steps"=w422, "Y2 data in"=w428, "X data in"=w430, "Y1 data in"=w429, "Y3 data in"=w427, "error in (no error)"=w425) -> ("Array of clusters"=w426:cluster{"Y data in":dbl[], "X data in":dbl[]}[], "error out"=w424:errorcluster)  [unwired: 1 in]
        n139 = local write "I vs Vd"(w426) -> ()
        n140 = call "4155C Config Chart Colours.vi"("Numeric"=w422, "XY Graph 2"=w423) -> ()  [unwired: 6 in]
        n141 = Open/Create/Replace File(file path (use dialog)=w480, error in=w424, operation (0:open)=w437) -> (refnum out=w490:refnum<file>, error out=w491:errorcluster)  [unwired: 3 in, 1 out]
        n142 = call "4155C Make Big 2d array.vi"("1D Var1"=w430, "1d IS"=w429, "1d ID"=w428, "1d IG"=w427, "1d SMU4"=w438, "SMU4"=w439, "VAR2 START"=w440, "Number of VAR2 steps"=w422, "VAR2 STEP"=w442, "VAR1 Name"="Vd", "Decimal places in header"=i8 1, "VAR2 Name"="Vg") -> ("Header array"=w486:string[], "Data array"=w487:dbl[][])  [unwired: 14 in]
        n143 = call "4155C Write array to file.vi"("Byte Stream File Refnum"=w490, "Header"=w486, "Data Array"=w487, "error in (no error)"=w491) -> ("dup refnum"=w488:refnum<file>, "error out"=w489:errorcluster)  [unwired: 1 in]
        n144 = Close File(refnum=w488, error in=w489) -> (error out=w475:errorcluster)  [unwired: 1 out]
      }
      frame "output-fpp" {
        n145 = Number To Decimal String(number=w500) -> (decimal integer string=w554:string)  [unwired: 1 in]
        n146 = Bundle By Name(cluster=w530, "Emergency Stop"=w557) -> (w567:T6)
        n147 = Delete From Array(array=w545, index=0 ("Index")) -> (deleted portion=w543:string, array with subset deleted=w542:string[])  [unwired: 1 in]
        n148 = VISA Write(VISA resource name=w521, write buffer=":PAGE:CHAN:MODE SWE;" ("write buffer (\"\")"), error in (no error)=w518) -> (VISA resource name out=w520:refnum<visa-resource-name>, error out=w519:errorcluster)  [unwired: 1 out]
        n149 = Concatenate Strings(w553, "-outputfpp-" ("Substring"), w554, w499, ".txt" ("Substring")) -> (w556:string)
        n150 = case shown="\"d\", Default" w543 {
          tunnel: [w568 w569] -> w541
          frame "s" {
            w568 = u16 0 items=["Single", "Double"] ("sweep mode")
          }
          frame "d", Default {
            w569 = u16 1 items=["Single", "Double"] ("sweep mode")
          }
        }
        n151 = Fract/Exp String To Number(string=w542) -> (number=w524:dbl[])  [unwired: 3 in, 1 out]
        n152 = String To Path(string=w556) -> (path=w552:path)
        n153 = Index Array(array=w524, index #1=0 ("Index")) -> (element #1=w540:dbl, element #2=w539:dbl, element #3=w538:dbl)  [unwired: 2 in]
        n154 = Delete From Array(array=w524, length=3 ("Length"), index=0 ("Index")) -> (array with subset deleted=w523:dbl[])  [unwired: 1 out]
        n155 = Bundle By Name(cluster=w532, "Gate Start"=w540, "Gate Stop"=w539, "Gate Step (linear only)"=w538, "Gate Compliance"=w550, "Range mode"=w516, "Range"=w515) -> (w566:T3)
        n156 = Index Array(array=w523, index #1=0 ("Index")) -> (element #1=w535:dbl, element #2=w534:dbl, element #3=w533:dbl)  [unwired: 2 in]
        n157 = call <vilib>:"compatOverwrite.vi"("overwrite (F)"=TRUE) -> ("overwrite?"=w504:T7)
        n158 = Bundle By Name(cluster=w531, "Drain Start"=w535, "Drain Stop"=w534, "Drain Step"=w533, "Drain Compliance"=w551, "Range mode"=w514, "Range"=w517) -> (w565:T4)
        n159 = call "4155C Output-FPP.vi"("VISA resource name in"=w520, "Gate"=w566, "Drain"=w565, "Timings"=w549, "error in (no error)"=w519, "sweep mode"=w541, "Panel controls"=w567) -> ("VD"=w509:dbl[], "Outparams"=w512:T8, "VISA Resource Name out"=w547:refnum<visa-resource-name>, "Vprobe2"=w508:dbl[], "ID"=w507:dbl[], "IG"=w506:dbl[], "Vprobe1"=w505:dbl[], "error out"=w548:errorcluster)  [unwired: 13 in]
        n160 = Unbundle By Name(w512) -> ("V2 Step"=w513:dbl, "V2 Start"=w511:dbl, "Number of points"=w510:i32)
        n161 = Open/Create/Replace File(file path (use dialog)=w552, error in=w548, operation (0:open)=w504) -> (refnum out=w562:refnum<file>, error out=w563:errorcluster)  [unwired: 3 in, 1 out]
        n162 = call "4155C Make Big 2d array FPP.vi"("1D Var1"=w509, "1d ID"=w507, "1d Vp2"=w508, "1d IG"=w506, "1d Vp1"=w505, "VAR2 START"=w511, "Number of VAR2 steps"=w510, "VAR2 STEP"=w513, "VAR1 Name"="Vd", "Decimal places in header"=i8 1, "VAR2 Name"="Vg") -> ("Header array"=w558:string[], "Data array"=w559:dbl[][])  [unwired: 15 in]
        n163 = call "4155C Write array to file.vi"("Byte Stream File Refnum"=w562, "Header"=w558, "Data Array"=w559, "error in (no error)"=w563) -> ("dup refnum"=w560:refnum<file>, "error out"=w561:errorcluster)  [unwired: 1 in]
        n164 = Close File(refnum=w560, error in=w561) -> (error out=w546:errorcluster)  [unwired: 1 out]
      }
      frame "itime" {
        n165 = Delete From Array(array=w584, index=0 ("Index")) -> (deleted portion=w585:string)  [unwired: 1 in, 1 out]
        n166 = case shown="\"l\"" w585 {
          tunnel: w583 -> [w589 w591 w594]
          tunnel: [w588 w590 w593] -> w576
          frame "s" {
            w587 = u32 0 items=["short  ", "medium  ", "long  "] ("integration time 2")
            n167 = Bundle By Name(cluster=w589, "integration time"=w587) -> (w588:T5)
          }
          frame "m", Default {
            w592 = u32 1 items=["short  ", "medium  ", "long  "] ("integration time 2")
            n168 = Bundle By Name(cluster=w591, "integration time"=w592) -> (w590:T5)
          }
          frame "l" {
            w595 = u32 2 items=["short  ", "medium  ", "long  "] ("integration time 2")
            n169 = Bundle By Name(cluster=w594, "integration time"=w595) -> (w593:T5)
          }
        }
      }
      frame "pulsed" {
        n170 = Delete From Array(array=w611, index=0 ("Index")) -> (deleted portion=w612:string, array with subset deleted=w599:string[])  [unwired: 1 in]
        n171 = case shown="\"on\", Default" w612 {
          tunnel: w610 -> [w622 w625]
          tunnel: [w621 w624] -> w603
          tunnel: w599 -> [w619 _]
          frame "on", Default {
            w620 = u16 1 items=["Continuous", "Pulsed"] ("sweep method")
            n172 = Fract/Exp String To Number(string=w619) -> (number=w617:dbl[])  [unwired: 3 in, 1 out]
            n173 = Index Array(array=w617, index #1=0 ("Index")) -> (element #1=w616:dbl, element #2=w615:dbl, element #3=w614:dbl)  [unwired: 2 in]
            n174 = Bundle By Name(cluster=w622, "sweep method"=w620, "Pulse period"=w616, "Base voltage"=w615, "Pulse width"=w614) -> (w621:T5)
          }
          frame "off" {
            w623 = u16 0 items=["Continuous", "Pulsed"] ("sweep method")
            n175 = Bundle By Name(cluster=w625, "sweep method"=w623) -> (w624:T5)
          }
        }
      }
      frame "gaterangemode" {
        n176 = Delete From Array(array=w639, index=0 ("Index")) -> (deleted portion=w640:string)  [unwired: 1 in, 1 out]
        n177 = case shown="\"f\"" w640 {
          tunnel: [w642 w643 w644] -> w629
          frame "a", Default {
            w642 = u16 0 items=["Auto", "Limited", "Fixed"] ("Gate Range\nmode 2")
          }
          frame "f" {
            w643 = u16 2 items=["Auto", "Limited", "Fixed"] ("Gate Range\nmode 2")
          }
          frame "l" {
            w644 = u16 1 items=["Auto", "Limited", "Fixed"] ("Gate Range\nmode 2")
          }
        }
      }
      frame "gaterange" {
        (unwired) u8 11 items=["10fA  ", "100fA  ", "1nA  ", "10nA", "100nA", "1uA", "10uA", "100uA", "1mA", "10mA", "100mA", "1A"] ("Gate Range 2")
        n178 = Delete From Array(array=w665, index=0 ("Index")) -> (deleted portion=w655:string)  [unwired: 1 in, 1 out]
        n179 = Scan Value(string=w655, format string="") -> (value=w653:dbl)  [unwired: 1 in, 1 out]
        n180 = Logarithm Base 10(1:w653) -> (0:w652:dbl)
        n181 = Round To Nearest(number=w652) -> (nearest integer value=w651:dbl)
        n182 = Add(x=w651, y=11.0) -> (x+y=w649:dbl)
        n183 = To Unsigned Byte Integer(number=w649) -> (unsigned 8bit integer=w648:u8)
      }
      frame "drainrange" {
        (unwired) u8 11 items=["10fA  ", "100fA  ", "1nA  ", "10nA", "100nA", "1uA", "10uA", "100uA", "1mA", "10mA", "100mA", "1A"] ("Gate Range 2")
        n184 = Delete From Array(array=w687, index=0 ("Index")) -> (deleted portion=w678:string)  [unwired: 1 in, 1 out]
        n185 = Scan Value(string=w678, format string="") -> (value=w676:dbl)  [unwired: 1 in, 1 out]
        n186 = Logarithm Base 10(1:w676) -> (0:w675:dbl)
        n187 = Round To Nearest(number=w675) -> (nearest integer value=w674:dbl)
        n188 = Add(x=w674, y=11.0) -> (x+y=w672:dbl)
        n189 = To Unsigned Byte Integer(number=w672) -> (unsigned 8bit integer=w671:u8)
      }
      frame "drainrangemode" {
        n190 = Delete From Array(array=w702, index=0 ("Index")) -> (deleted portion=w703:string)  [unwired: 1 in, 1 out]
        n191 = case shown="\"f\"" w703 {
          tunnel: [w705 w706 w707] -> w692
          frame "a", Default {
            w705 = u16 0 items=["Auto", "Limited", "Fixed"] ("Gate Range\nmode 2")
          }
          frame "f" {
            w706 = u16 2 items=["Auto", "Limited", "Fixed"] ("Gate Range\nmode 2")
          }
          frame "l" {
            w707 = u16 1 items=["Auto", "Limited", "Fixed"] ("Gate Range\nmode 2")
          }
        }
      }
      frame "Error", Default {
      }
      frame "logfile" {
        n192 = Number To Decimal String(number=w724) -> (decimal integer string=w759:string)  [unwired: 1 in]
        n193 = Concatenate Strings(w758, "logfile" ("Substring"), w759, w722, ".txt" ("Substring")) -> (w756:string)
        n194 = String To Path(string=w756) -> (path=w729:path)
        n195 = Unbundle(w755) -> ("integration time"=w754:u32, "Short/Long integration time"=w753:dbl, "hold time (sec)"=w752:dbl, "delay time (sec)"=w751:dbl, "Step Time (0 disables)"=w750:dbl, "sweep method"=w749:u16, "Pulse period"=w748:dbl, "Base voltage"=w747:dbl, "Pulse width"=w746:dbl)
        n196 = Build Array(w754, w753, w752, w751, w750, w749, w748, w747, w746, w740, w741, w742, w743, w744, w745) -> (w733:dbl[])
        n197 = Insert Into Array(array=dbl[][] [] ("Input Array"), new element=w733) -> (w732:dbl[][])  [unwired: 2 in]
        n198 = call <vilib>:"compatOverwrite.vi"("overwrite (F)"=TRUE) -> ("overwrite?"=w727:T7)
        n199 = Open/Create/Replace File(file path (use dialog)=w729, error in=w731, operation (0:open)=w727) -> (refnum out=w737:refnum<file>, error out=w736:errorcluster)  [unwired: 3 in, 1 out]
        n200 = call "4155C Write array to file.vi"("Byte Stream File Refnum"=w737, "Header"=string[] ["Int Time", "Short/Long Itime", "Hold time", "Delay time", "Step time", "Sweep method", "Pulse period", "Base Voltage", "Pulse width", "Drain compliance", "Gate compliance", "Gate range mode", "Gate range", "S/D range mode", "S/D range"], "Data Array"=w732, "error in (no error)"=w736) -> ("dup refnum"=w739:refnum<file>, "error out"=w738:errorcluster)  [unwired: 1 in]
        n201 = Close File(refnum=w739, error in=w738) -> (error out=w730:errorcluster)  [unwired: 1 out]
      }
      frame "sample" {
        n202 = Number To Decimal String(number=w764) -> (decimal integer string=w812:string)  [unwired: 1 in]
        n203 = Fract/Exp String To Number(string=w809) -> (number=w770:dbl[])  [unwired: 3 in, 1 out]
        n204 = Concatenate Strings(w787, "-sample-" ("Substring"), w812, w762, ".txt" ("Substring")) -> (w810:string)
        n205 = String To Path(string=w810) -> (path=w791:path)
        n206 = Index Array(array=w770, index=0 ("Index")) -> (element=w807:dbl)
        n207 = Index Array(array=w770, index=2 ("Index")) -> (element=w803:dbl)
        n208 = Index Array(array=w770, index=3 ("Index")) -> (element=w772:dbl)
        n209 = Index Array(array=w770, index=4 ("Index")) -> (element=w769:dbl)
        n210 = call "4155C Config Sampling Measurements.vi"("Sampling interval"=w769, "Sample time"=w772, "Display on/off"=TRUE, "Timings"=w778, "Num Points"=w803, "error in (no error)"=w814, "Drain Compliance"=w813, "Gate Compliance"=w788, "VISA session"=w815) -> ("error out"=w816:errorcluster, "dup VISA resource name"=w817:refnum<visa-resource-name>)  [unwired: 1 in]
        n211 = Index Array(array=w770, index=1 ("Index")) -> (element=w804:dbl)
        n212 = call "4155C Take Sample.vi"("Emergency Stop"=w784, "error in (no error)"=w816, "Vd"=w804, "Vg"=w807, "VISA resource name in"=w817) -> ("error out"=w782:errorcluster, "Id"=w819:dbl[], "Ig"=w793:dbl[], "VISA Resource Name out"=w780:refnum<visa-resource-name>, "Is"=w818:dbl[], "Time"=w797:dbl[])  [unwired: 1 in]
        n213 = Insert Into Array(array=dbl[][] [] ("Input Array"), new element=w797) -> (w796:dbl[][])  [unwired: 2 in]
        n214 = Insert Into Array(array=w796, new element=w793) -> (w795:dbl[][])  [unwired: 2 in]
        n215 = Insert Into Array(array=w795, new element=w819) -> (w794:dbl[][])  [unwired: 2 in]
        n216 = VISA Write(VISA resource name=w780, write buffer=":DISP ON" ("write buffer (\"\")"), error in (no error)=w782) -> (VISA resource name out=w779:refnum<visa-resource-name>, error out=w781:errorcluster)  [unwired: 1 out]
        n217 = Insert Into Array(array=w794, new element=w818) -> (w786:dbl[][])  [unwired: 2 in]
        n218 = Transpose 2D Array(2D array=w786) -> (transposed array=w785:dbl[][])
        n219 = call <vilib>:"compatOverwrite.vi"("overwrite (F)"=TRUE) -> ("overwrite?"=w767:T7)
        n220 = Open/Create/Replace File(file path (use dialog)=w791, error in=w781, operation (0:open)=w767) -> (refnum out=w800:refnum<file>, error out=w799:errorcluster)  [unwired: 3 in, 1 out]
        n221 = call "4155C Write array to file.vi"("Byte Stream File Refnum"=w800, "Header"=string[] ["Time /s", "Ig /A", "Id /A", "Is /A"], "Data Array"=w785, "error in (no error)"=w799) -> ("dup refnum"=w802:refnum<file>, "error out"=w801:errorcluster)  [unwired: 1 in]
        n222 = Close File(refnum=w802, error in=w801) -> (error out=w789:errorcluster)  [unwired: 1 out]
      }
      frame "samplei" {
        n223 = Number To Decimal String(number=w822) -> (decimal integer string=w874:string)  [unwired: 1 in]
        n224 = Fract/Exp String To Number(string=w871) -> (number=w838:dbl[])  [unwired: 3 in, 1 out]
        n225 = Concatenate Strings(w853, "-samplei-" ("Substring"), w874, w821, ".txt" ("Substring")) -> (w872:string)
        n226 = String To Path(string=w872) -> (path=w856:path)
        n227 = Index Array(array=w838, index=4 ("Index")) -> (element=w832:dbl)
        n228 = Index Array(array=w838, index=3 ("Index")) -> (element=w833:dbl)
        n229 = Index Array(array=w838, index=1 ("Index")) -> (element=w835:dbl)
        n230 = Index Array(array=w838, index=0 ("Index")) -> (element=w836:dbl)
        n231 = Index Array(array=w838, index=2 ("Index")) -> (element=w834:dbl)
        n232 = call "4155C Config SamplingI Measurements.vi"("Sample time"=w834, "Display on/off"=TRUE, "Timings"=w845, "Num Points"=w835, "error in (no error)"=w876, "Sampling interval"=w833, "VISA session"=w877) -> ("error out"=w878:errorcluster, "dup VISA resource name"=w879:refnum<visa-resource-name>)  [unwired: 3 in]
        n233 = call "4155C Take SampleI.vi"("Emergency Stop"=w850, "error in (no error)"=w878, "Idg 2"=w836, "Vdg compliance 2"=w832, "VISA resource name in"=w879) -> ("error out"=w848:errorcluster, "Idg"=w881:dbl[], "Vdg"=w858:dbl[], "VISA Resource Name out"=w846:refnum<visa-resource-name>, "Is"=w880:dbl[], "Time"=w862:dbl[])  [unwired: 1 in]
        n234 = Insert Into Array(array=dbl[][] [] ("Input Array"), new element=w862) -> (w861:dbl[][])  [unwired: 2 in]
        n235 = Insert Into Array(array=w861, new element=w858) -> (w860:dbl[][])  [unwired: 2 in]
        n236 = Insert Into Array(array=w860, new element=w881) -> (w859:dbl[][])  [unwired: 2 in]
        n237 = VISA Write(VISA resource name=w846, write buffer=":DISP ON" ("write buffer (\"\")"), error in (no error)=w848) -> (VISA resource name out=w831:refnum<visa-resource-name>, error out=w847:errorcluster)  [unwired: 1 out]
        n238 = Insert Into Array(array=w859, new element=w880) -> (w852:dbl[][])  [unwired: 2 in]
        n239 = Transpose 2D Array(2D array=w852) -> (transposed array=w851:dbl[][])
        n240 = call <vilib>:"compatOverwrite.vi"("overwrite (F)"=TRUE) -> ("overwrite?"=w826:T7)
        n241 = Open/Create/Replace File(file path (use dialog)=w856, error in=w847, operation (0:open)=w826) -> (refnum out=w865:refnum<file>, error out=w864:errorcluster)  [unwired: 3 in, 1 out]
        n242 = call "4155C Write array to file.vi"("Byte Stream File Refnum"=w865, "Header"=string[] ["Time /s", "Vdg /V", "Idg /A", "Is /A"], "Data Array"=w851, "error in (no error)"=w864) -> ("dup refnum"=w867:refnum<file>, "error out"=w866:errorcluster)  [unwired: 1 in]
        n243 = Close File(refnum=w867, error in=w866) -> (error out=w829:errorcluster)  [unwired: 1 out]
        n244 = VISA Write(VISA resource name=w831, write buffer=";:PAGE:SCON:STAN OFF;:PAGE:CHAN:VSU2:DIS;" ("write buffer (\"\")"), error in (no error)=w829) -> (VISA resource name out=w827:refnum<visa-resource-name>, error out=w828:errorcluster)  [unwired: 1 out]
      }
      frame "#" {
        n245 = VISA Write(VISA resource name=w889, write buffer=":DISP ON" ("write buffer (\"\")"), error in (no error)=w888) -> (VISA resource name out=w887:refnum<visa-resource-name>, error out=w886:errorcluster)  [unwired: 1 out]
      }
      frame "stressV" {
        n246 = Number To Decimal String(number=w900) -> (decimal integer string=w941:string)  [unwired: 1 in]
        n247 = Fract/Exp String To Number(string=w938) -> (number=w911:dbl[])  [unwired: 3 in, 1 out]
        n248 = Concatenate Strings(w925, "-stressV-" ("Substring"), w941, w899, ".txt" ("Substring")) -> (w939:string)
        n249 = String To Path(string=w939) -> (path=w929:path)
        n250 = Index Array(array=w911, index=3 ("Index")) -> (element=w908:dbl)
        n251 = Index Array(array=w911, index=1 ("Index")) -> (element=w906:dbl)
        n252 = Index Array(array=w911, index=0 ("Index")) -> (element=w905:dbl)
        n253 = Index Array(array=w911, index=4 ("Index")) -> (element=w910:dbl)
        n254 = Index Array(array=w911, index=2 ("Index")) -> (element=w907:dbl)
        n255 = call "4155C Config V Stress.vi"("VISA session"=w944, "ID compliance"=w908, "VD"=w906, "VG"=w905, "IG compliance"=w907, "error in (no error)"=w943, "Display on/off"=TRUE) -> ("dup VISA resource name"=w946:refnum<visa-resource-name>, "error out"=w945:errorcluster)
        n256 = call "4155C Apply Stress.vi"("error in (no error)"=w945, "Duration"=w910, "Emergency Stop"=w924, "VISA resource name in"=w946) -> ("error out"=w922:errorcluster, "VISA Resource Name out"=w920:refnum<visa-resource-name>)
        n257 = VISA Write(VISA resource name=w920, write buffer=":DISP ON" ("write buffer (\"\")"), error in (no error)=w922) -> (VISA resource name out=w919:refnum<visa-resource-name>, error out=w921:errorcluster)  [unwired: 1 out]
        n258 = call <vilib>:"compatOverwrite.vi"("overwrite (F)"=TRUE) -> ("overwrite?"=w904:T7)
        n259 = Open/Create/Replace File(file path (use dialog)=w929, error in=w921, operation (0:open)=w904) -> (refnum out=w932:refnum<file>, error out=w931:errorcluster)  [unwired: 3 in, 1 out]
        n260 = call "4155C Write array to file.vi"("Byte Stream File Refnum"=w932, "Header"=string[] ["V stress completed successfully", ""], "error in (no error)"=w931) -> ("dup refnum"=w934:refnum<file>, "error out"=w933:errorcluster)  [unwired: 2 in]
        n261 = Close File(refnum=w934, error in=w933) -> (error out=w927:errorcluster)  [unwired: 1 out]
      }
      frame "stressI" {
        n262 = Number To Decimal String(number=w949) -> (decimal integer string=w986:string)  [unwired: 1 in]
        n263 = Fract/Exp String To Number(string=w983) -> (number=w958:dbl[])  [unwired: 3 in, 1 out]
        n264 = Concatenate Strings(w970, "-stressI-" ("Substring"), w986, w948, ".txt" ("Substring")) -> (w984:string)
        n265 = String To Path(string=w984) -> (path=w974:path)
        n266 = Index Array(array=w958, index=1 ("Index")) -> (element=w954:dbl)
        n267 = Index Array(array=w958, index=0 ("Index")) -> (element=w955:dbl)
        n268 = call "4155C Config I Stress.vi"("VISA session"=w989, "IDG"=w955, "VDG compliance"=w954, "error in (no error)"=w988, "Display on/off"=TRUE) -> ("dup VISA resource name"=w991:refnum<visa-resource-name>, "error out"=w990:errorcluster)
        n269 = Index Array(array=w958, index=2 ("Index")) -> (element=w956:dbl)
        n270 = call "4155C Apply Stress.vi"("error in (no error)"=w990, "Duration"=w956, "Emergency Stop"=w969, "VISA resource name in"=w991) -> ("error out"=w967:errorcluster, "VISA Resource Name out"=w965:refnum<visa-resource-name>)
        n271 = VISA Write(VISA resource name=w965, write buffer=":DISP ON" ("write buffer (\"\")"), error in (no error)=w967) -> (VISA resource name out=w964:refnum<visa-resource-name>, error out=w966:errorcluster)  [unwired: 1 out]
        n272 = call <vilib>:"compatOverwrite.vi"("overwrite (F)"=TRUE) -> ("overwrite?"=w953:T7)
        n273 = Open/Create/Replace File(file path (use dialog)=w974, error in=w966, operation (0:open)=w953) -> (refnum out=w977:refnum<file>, error out=w976:errorcluster)  [unwired: 3 in, 1 out]
        n274 = call "4155C Write array to file.vi"("Byte Stream File Refnum"=w977, "Header"=string[] ["I stress completed successfully", ""], "error in (no error)"=w976) -> ("dup refnum"=w979:refnum<file>, "error out"=w978:errorcluster)  [unwired: 2 in]
        n275 = Close File(refnum=w979, error in=w978) -> (error out=w972:errorcluster)  [unwired: 1 out]
      }
      frame "vsu2pulse" {
        n276 = Number To Decimal String(number=w994) -> (decimal integer string=w1029:string)  [unwired: 1 in]
        n277 = Fract/Exp String To Number(string=w1026) -> (number=w1002:dbl[])  [unwired: 3 in, 1 out]
        n278 = Concatenate Strings(w1014, "-vsu2-" ("Substring"), w1029, w993, ".txt" ("Substring")) -> (w1027:string)
        n279 = String To Path(string=w1027) -> (path=w1018:path)
        n280 = Index Array(array=w1002, index=1 ("Index")) -> (element=w1001:dbl)
        n281 = Index Array(array=w1002, index=0 ("Index")) -> (element=w999:dbl)
        n282 = call "4155C Config VSU2 Stress.vi"("error in (no error)"=w1031, "VSU2"=w999, "Display on/off"=TRUE, "VISA session"=w1032) -> ("error out"=w1033:errorcluster, "dup VISA resource name"=w1034:refnum<visa-resource-name>)
        n283 = call "4155C Apply Stress.vi"("error in (no error)"=w1033, "Duration"=w1001, "Emergency Stop"=w1013, "VISA resource name in"=w1034) -> ("error out"=w1011:errorcluster, "VISA Resource Name out"=w1009:refnum<visa-resource-name>)
        n284 = VISA Write(VISA resource name=w1009, write buffer=":DISP ON" ("write buffer (\"\")"), error in (no error)=w1011) -> (VISA resource name out=w1008:refnum<visa-resource-name>, error out=w1010:errorcluster)  [unwired: 1 out]
        n285 = call <vilib>:"compatOverwrite.vi"("overwrite (F)"=TRUE) -> ("overwrite?"=w998:T7)
        n286 = Open/Create/Replace File(file path (use dialog)=w1018, error in=w1010, operation (0:open)=w998) -> (refnum out=w1021:refnum<file>, error out=w1020:errorcluster)  [unwired: 3 in, 1 out]
        n287 = call "4155C Write array to file.vi"("Byte Stream File Refnum"=w1021, "Header"=string[] ["VSU2 pulse completed successfully", ""], "error in (no error)"=w1020) -> ("dup refnum"=w1023:refnum<file>, "error out"=w1022:errorcluster)  [unwired: 2 in]
        n288 = Close File(refnum=w1023, error in=w1022) -> (error out=w1016:errorcluster)  [unwired: 1 out]
      }
      frame "sample-fpp" {
        w1048 = string[] ["Time /s", "Id VgVd /A", "Ig VgVd /A", "Vp1 VgVd /V", "Vp2 VgVd /V"] ("Header")
        w1052 = "%d" ("format string")
        n289 = Number To Decimal String(number=w1037) -> (decimal integer string=w1100:string)  [unwired: 1 in]
        n290 = Fract/Exp String To Number(string=w1097) -> (number=w1085:dbl[])  [unwired: 3 in, 1 out]
        n291 = Concatenate Strings(w1091, "-samplefpp-" ("Substring"), w1100, w1036, ".txt" ("Substring")) -> (w1098:string)
        n292 = String To Path(string=w1098) -> (path=w1060:path)
        n293 = Index Array(array=w1085, index=0 ("Index")) -> (element=w1046:dbl)
        n294 = Index Array(array=w1085, index=1 ("Index")) -> (element=w1045:dbl)
        n295 = Index Array(array=w1085, index=2 ("Index")) -> (element=w1093:dbl)
        n296 = Index Array(array=w1085, index=3 ("Index")) -> (element=w1083:dbl)
        n297 = call "4155C Config Sampling Measurements FPP.vi"("VISA session"=w1103, "Num Points"=w1093, "Vg"=w1046, "Display on/off"=TRUE, "Gate Compliance"=w1092, "Drain Compliance"=w1101, "Standby"="Standby", "error in (no error)"=w1102, "Timings"=w1090, "Vd"=w1045, "Sample time"=w1083) -> ("dup VISA resource name"=w1062:refnum<visa-resource-name>, "error out"=w1061:errorcluster)  [unwired: 3 in]
        n298 = Number To Decimal String(number=w1046) -> (decimal integer string=w1072:string)  [unwired: 1 in]
        n299 = call "4155C Take Sample FPP.vi"("VISA resource name in"=w1062, "error in (no error)"=w1061, "Emergency Stop"=w1063) -> ("Time"=w1067:dbl[], "Vp1"=w1077:dbl[], "VISA Resource Name out"=w1043:refnum<visa-resource-name>, "Ig"=w1065:dbl[], "Id"=w1066:dbl[], "Vp2"=w1075:dbl[], "error out"=w1064:errorcluster)  [unwired: 10 in]
        n300 = Insert Into Array(array=dbl[][] [] ("Input Array"), new element=w1067) -> (w1081:dbl[][])  [unwired: 2 in]
        n301 = Number To Decimal String(number=w1045) -> (decimal integer string=w1070:string)  [unwired: 1 in]
        n302 = Insert Into Array(array=w1081, new element=w1066) -> (w1080:dbl[][])  [unwired: 2 in]
        n303 = Concatenate Strings("(Vg = " ("Substring"), w1072, "V, Vd = " ("Substring"), w1070, "V)" ("Substring")) -> (w1068:string)
        n304 = Insert Into Array(array=w1080, new element=w1065) -> (w1079:dbl[][])  [unwired: 2 in]
        n305 = Insert Into Array(array=w1079, new element=w1077) -> (w1076:dbl[][])  [unwired: 2 in]
        n306 = Insert Into Array(array=w1076, new element=w1075) -> (w1044:dbl[][])  [unwired: 2 in]
        n307 = call <vilib>:"compatOverwrite.vi"("overwrite (F)"=TRUE) -> ("overwrite?"=w1041:T7)
        n308 = Open/Create/Replace File(file path (use dialog)=w1060, error in=w1064, operation (0:open)=w1041) -> (refnum out=w1057:refnum<file>, error out=w1058:errorcluster)  [unwired: 3 in, 1 out]
        n309 = Array To Spreadsheet String(array=w1048, 3:w1052) -> (spreadsheet string=w1054:string)  [unwired: 1 in]
        n310 = Transpose 2D Array(2D array=w1044) -> (transposed array=w1074:dbl[][])
        n311 = Search and Replace String(replace all?=TRUE ("replace all? (F)"), input string=w1054, search string="VgVd", replace string=w1068) -> (result string=w1050:string)  [unwired: 4 in, 3 out]
        n312 = Spreadsheet String To Array(format string=w1052, spreadsheet string=w1050, array type (2D Dbl)=w1048) -> (array=w1049:string[])  [unwired: 1 in]
        n313 = call "4155C Write array to file.vi"("Byte Stream File Refnum"=w1057, "Header"=w1049, "Data Array"=w1074, "error in (no error)"=w1058) -> ("dup refnum"=w1055:refnum<file>, "error out"=w1056:errorcluster)  [unwired: 1 in]
        n314 = Close File(refnum=w1055, error in=w1056) -> (error out=w1042:errorcluster)  [unwired: 1 out]
      }
      frame "resample-fpp" {
        w1119 = string[] ["Time /s", "Id VgVd /A", "Ig VgVd /A", "Vp1 VgVd /V", "Vp2 VgVd /V"] ("Header")
        w1123 = "%d" ("format string")
        n315 = Number To Decimal String(number=w1105) -> (decimal integer string=w1163:string)  [unwired: 1 in]
        n316 = Fract/Exp String To Number(string=w1160) -> (number=w1112:dbl[])  [unwired: 3 in, 1 out]
        n317 = Concatenate Strings(w1156, "-resamplefpp-" ("Substring"), w1163, w1106, ".txt" ("Substring")) -> (w1161:string)
        n318 = String To Path(string=w1161) -> (path=w1131:path)
        n319 = Index Array(array=w1112, index=0 ("Index")) -> (element=w1118:dbl)
        n320 = Index Array(array=w1112, index=1 ("Index")) -> (element=w1117:dbl)
        n321 = Number To Decimal String(number=w1118) -> (decimal integer string=w1141:string)  [unwired: 1 in]
        n322 = call "4155C Take Sample FPP.vi"("VISA resource name in"=w1114, "error in (no error)"=w1113, "Emergency Stop"=w1132) -> ("Time"=w1136:dbl[], "Vp1"=w1146:dbl[], "VISA Resource Name out"=w1116:refnum<visa-resource-name>, "Ig"=w1134:dbl[], "Id"=w1135:dbl[], "Vp2"=w1144:dbl[], "error out"=w1133:errorcluster)  [unwired: 10 in]
        n323 = Insert Into Array(array=dbl[][] [] ("Input Array"), new element=w1136) -> (w1150:dbl[][])  [unwired: 2 in]
        n324 = Number To Decimal String(number=w1117) -> (decimal integer string=w1139:string)  [unwired: 1 in]
        n325 = Insert Into Array(array=w1150, new element=w1135) -> (w1149:dbl[][])  [unwired: 2 in]
        n326 = Concatenate Strings("(Vg = " ("Substring"), w1141, "V, Vd = " ("Substring"), w1139, "V)" ("Substring")) -> (w1137:string)
        n327 = Insert Into Array(array=w1149, new element=w1134) -> (w1148:dbl[][])  [unwired: 2 in]
        n328 = Insert Into Array(array=w1148, new element=w1146) -> (w1145:dbl[][])  [unwired: 2 in]
        n329 = Insert Into Array(array=w1145, new element=w1144) -> (w1111:dbl[][])  [unwired: 2 in]
        n330 = call <vilib>:"compatOverwrite.vi"("overwrite (F)"=TRUE) -> ("overwrite?"=w1110:T7)
        n331 = Open/Create/Replace File(file path (use dialog)=w1131, error in=w1133, operation (0:open)=w1110) -> (refnum out=w1128:refnum<file>, error out=w1129:errorcluster)  [unwired: 3 in, 1 out]
        n332 = Array To Spreadsheet String(array=w1119, 3:w1123) -> (spreadsheet string=w1125:string)  [unwired: 1 in]
        n333 = Transpose 2D Array(2D array=w1111) -> (transposed array=w1143:dbl[][])
        n334 = Search and Replace String(replace all?=TRUE ("replace all? (F)"), input string=w1125, search string="VgVd", replace string=w1137) -> (result string=w1121:string)  [unwired: 4 in, 3 out]
        n335 = Spreadsheet String To Array(format string=w1123, spreadsheet string=w1121, array type (2D Dbl)=w1119) -> (array=w1120:string[])  [unwired: 1 in]
        n336 = call "4155C Write array to file.vi"("Byte Stream File Refnum"=w1128, "Header"=w1120, "Data Array"=w1143, "error in (no error)"=w1129) -> ("dup refnum"=w1126:refnum<file>, "error out"=w1127:errorcluster)  [unwired: 1 in]
        n337 = Close File(refnum=w1126, error in=w1127) -> (error out=w1115:errorcluster)  [unwired: 1 out]
      }
      frame "serial" {
        n338 = Index Array(array=w1168, index=0 ("Index")) -> (element=w1167:string)
        n339 = call "Serial write and read v0.4.vi"("Termination char\n(0xA = '\\n' = LF)\n(0xD = '\\r' = CR)"="Termination char\n(0xA = '\\n' = LF)\n(0xD = '\\r' = CR)", "Enable Termination\nChar (T)"="Enable Termination\nChar (T)", "parity"="parity", "stop bits"="stop bits", "string to write"=w1167, "flow control"="flow control", "byte count"="byte count", "Serial Settings:Serial End Mode for Reads"="Serial Settings:Serial End Mode for Reads", "Timeout (ms)"="Timeout (ms)", "error in (no error)"=w1173, "VISA resource name"="VISA resource name", "baud rate"="baud rate", "data bits"="data bits") -> ("read string"=→"Serial port output":string, "error out"=w1172:errorcluster)  [unwired: 1 in]
      }
    }
    n340 = Build Array("Time /s" ("element"), "Id max /A" ("VAR2 Name"), "Id min /A" ("VAR2 Name")) -> (w64:string[])
    n341 = Build Array(w59, w58, w50) -> (w57:dbl[][])
    n342 = Transpose 2D Array(2D array=w57) -> (transposed array=w56:dbl[][])
    n343 = Concatenate Strings(w55, "-Ion-Ioff", ".txt" ("Suffix")) -> (w72:string)
    n344 = Array To Spreadsheet String(array=w64, 3:"" ("format string")) -> (spreadsheet string=w63:string)  [unwired: 1 in]
    n345 = Array To Spreadsheet String(array=w56, 3:"%e" ("format string")) -> (spreadsheet string=w62:string)  [unwired: 1 in]
    n346 = String To Path(string=w72) -> (path=w71:path)
    n347 = Build Array(w63, w62) -> (w61:string[])
    n348 = Write to Text File(file (use dialog)=w71, text=w61, error in=w53) -> (refnum out=w73:refnum<file>, error out=w60:errorcluster)  [unwired: 1 in, 1 out]
    n349 = Close File(refnum=w73, error in=w60) -> (error out=w52:errorcluster)  [unwired: 1 out]
    "Line running" <- w83
    "Total lines" <- w82
  }
  "error out" <- w1
